vi "ME_acquire_10_DeltaForce_mod.vi"() -> ()   [LabVIEW 2015]
doc: "Use this template to build a producer/consumer design pattern. Use this template when you need to execute a process, such as data analysis, when a data source, such as a triggered acquisition, produces data at an uneven rate and you need to execute the process when the data becomes available."
uses:
  oxford_driver/Oxford Drivers/BUSGEN.LLB/OxfordAddress.ctl
  <vilib>/express/express arith-compare/Formula/XNode/ExpressFormulaBlockNode.xnode
  Mode.ctl
  <vilib>/Utility/file.llb/Write Delimited Spreadsheet (DBL).vi
  <vilib>/Analysis/NI_AALBase.lvlib
  <vilib>/Analysis/baseanly.llb/Mean (DBL).vi
panel:
  out "deltaUaux":dbl
  out "Actual Voltage (V)":dbl caption="Actual AuxV" step=0.1
  out "remaining elements":T1(array[cluster])
  in  "Stop":bool
  out "SaveSweep":bool=TRUE
  out "Measurement File_dn":path
  out "Measurement File_up":path
  out "Measurement File_average":path
  out "Actual Polarization":dbl
  in  "Reset IB?":bool
  in  "First?":bool
  in  "Save Period":dbl=1.0
  out "Averaged I(B)":dbl[][](array[numeric])
  out "P(uC/mm^2)":dbl[](array[numeric])
  in  "Sweep":bool
  out "P(B)":cluster{"yi":dbl[], dbl[]}(graph)
  out "Offset array":dbl[](array[numeric])
  in  "stop 2":bool
  in  "dB":dbl=0.005
  in  "Dwell Time (ms)":u32=1
  out "appended array":dbl[][](array[numeric])
  out "Actual B Field (T)":dbl
  out "Actual Temperature (K)":dbl
  out "Actual Current (pA)":dbl
  in  "Tab Control":T2(tab)
  in  "Max temperature (K)":dbl=20.0
  in  "Min Temperature (K)":dbl=4.5
  out "P(T)":cluster{"yi":dbl[], dbl[]}(graph)
  out "I(T)":cluster{dbl[], dbl[]}(graph)
  in  "Set temperature (K)":dbl=4.5
  in  "Temp Ramping Rate (K/min)":dbl=10.0
  in  "Heater Range":enum16{"Off", "Low", "Medium", "High"}(ring)
  in  "Heater On/Off":bool
  out "Setpoint Temperature (K)":dbl
  in  "FileName":string
  out "Step Temp":bool
  out "j":i32
  out "i":i32
  in  "Max Countl":i32
  in  "Record ALL":bool
  in  "Sweep Rate Array":dbl[](array[numeric])=[2.0, 1.0, 0.5, 0.1, 0.05, 9.0, 10.0, 11.0, 12.0]
  out "I(B) 3":cluster{dbl[], dbl[]}[](graph)
  in  "Go to Set":bool
  in  "Set Field (T)":dbl
  in  "Field To Zero":bool
  in  "Sweep Rate (T/min)":dbl=2.0 format="%.6f"
  in  "Min Field (T)":dbl
  in  "Max Field (T)":dbl=0.15
  out "Up/Down":bool
  out "I(B) /Averaged/ 2":cluster{"B array":dbl[], dbl[]}[](graph)
  in  "Temperature Array":dbl[](array[numeric])=[4.5, 5.0, 6.0, 7.0, 8.0, 9.0, 10.0, 11.0, 12.0]
  out "New":bool=TRUE
  out "Step Rate":bool
  out "Finished":bool=TRUE
  in  "Directory":string
  out "Wait (s)":dbl
  in  "secs to wait":dbl=180.0
  in  "Max count array":i32[](array[numeric])=[2, 1, 0, 0, 0, 9, 10, 11, 12]
  out "Target Field":dbl
  in  "Measure Noise":bool
  in  "Cycles":i32
  in  "maximum value":dbl=10.0 format="%0.2f"
  in  "minimum value":dbl=-10.0 format="%0.2f"
  in  "physical channels":tag="Dev1/ai1"
  out "PSD (pA/Hz^1/2) Peaks Removed":cluster{"f0":dbl, "df":dbl, "magnitude":dbl[]}(graph)
  out "PSD (pA/Hz^1/2)":cluster{"f0":dbl, "df":dbl, "magnitude":dbl[]}(graph)
  out "Current (pA) Filtered":waveform(dbl)(graph)
  out "Current (pA)":dbl[](graph)
  in  "Samples per channel":i32=1000
  in  "Rate":dbl=1000.0 format="%0.2f"
  in  "Cut-Off Frequency":dbl=100.0 caption="Lower Cut-Off"
  in  "Filter On":bool
  in  "Lock_in_Amplifier":refnum<visa-resource-name>="GPIB0::5::INSTR"
  out "Dc offset":dbl
  in  "Calibrate":bool
  in  "IV converter":refnum<visa-resource-name>="GPIB0::20::INSTR"
  in  "Magnetic Field":refnum<visa-resource-name>="GPIB0::21::INSTR"
  out "Time Lag":dbl=0.0500025749206543
  in  "Lake Shore":refnum<visa-resource-name>="GPIB0::11::INSTR"
  in  "Temp Refresh (s)":dbl=0.1
  in  "Sampling rate (Hz)":dbl=10.0
  in  "Gain (V/A)":dbl=1000000000.0
  in  "Sample area (mm^2)":dbl=3.9
  out "B_V":cluster{dbl[], "Best Linear Fit":dbl[]}[](graph)=[{[-0.00854253601, 0.00626134724, 0.0219834428, 0.0379117736, 0.0535871506, 0.0694316728, 0.0851615152, 0.100816481, 0.116478038, 0.132148461, 0.147876163, 0.16341701, 0.178976744, 0.194563632, 0.210251739, 0.225738944, 0.241298253, 0.256806034, 0.272344374, 0.287933477, 0.303494709, 0.318997125, 0.334591297, 0.350146681, 0.365618053, 0.380940961, 0.39666457, 0.412213675, 0.427724671, 0.443221444, 0.458760641, 0.474360042, 0.489915118, 0.505330598, 0.520967119, 0.536347531, 0.551813711, 0.567441155, 0.582995861, 0.598507522, 0.614041988, 0.629563151, 0.645106262, 0.660611914, 0.676136149, 0.691553948, 0.7071244, 0.72262999, 0.738171137, 0.753700392, 0.76919513, 0.784778028, 0.800215944, 0.8156961, 0.831325434, 0.846852183, 0.862326812, 0.877819169, 0.893312568, 0.90888536, 0.924354789], "Best Linear Fit"=[0.0, 0.005, 0.01, 0.015, 0.02, 0.025, 0.03, 0.035, 0.04, 0.045, 0.05, 0.055, 0.06, 0.065, 0.07, 0.075, 0.08, 0.085, 0.09, 0.095, 0.1, 0.105, 0.11, 0.115, 0.12, 0.125, 0.13, 0.135, 0.14, 0.145, 0.15, 0.155, 0.16, 0.165, 0.17, 0.175, 0.18, 0.185, 0.19, 0.195, 0.2, 0.205, 0.21, 0.215, 0.22, 0.225, 0.23, 0.235, 0.24, 0.245, 0.25, 0.255, 0.26, 0.265, 0.27, 0.275, 0.28, 0.285, 0.29, 0.295, 0.3]}, {[-0.00854253601, 0.00626134724, 0.0219834428, 0.0379117736, 0.0535871506, 0.0694316728, 0.0851615152, 0.100816481, 0.116478038, 0.132148461, 0.147876163, 0.16341701, 0.178976744, 0.194563632, 0.210251739, 0.225738944, 0.241298253, 0.256806034, 0.272344374, 0.287933477, 0.303494709, 0.318997125, 0.334591297, 0.350146681, 0.365618053, 0.380940961, 0.39666457, 0.412213675, 0.427724671, 0.443221444, 0.458760641, 0.474360042, 0.489915118, 0.505330598, 0.520967119, 0.536347531, 0.551813711, 0.567441155, 0.582995861, 0.598507522, 0.614041988, 0.629563151, 0.645106262, 0.660611914, 0.676136149, 0.691553948, 0.7071244, 0.72262999, 0.738171137, 0.753700392, 0.76919513, 0.784778028, 0.800215944, 0.8156961, 0.831325434, 0.846852183, 0.862326812, 0.877819169, 0.893312568, 0.90888536, 0.924354789], "Best Linear Fit"=[-0.00022554388023060128, 0.004536267537808887, 0.009593430775915074, 0.014716931562355689, 0.01975906732634002, 0.024855610270593523, 0.029915265354287977, 0.03495083565949541, 0.03998852608757118, 0.045029068349812316, 0.05008803495326229, 0.055086897848955874, 0.060091835929837946, 0.06510550835596321, 0.07015173884687344, 0.07513334727738563, 0.08013814865293042, 0.08512637555172443, 0.0901244320467579, 0.09513881694893507, 0.10014423687592358, 0.10513073807087174, 0.11014675346564809, 0.1151502923271957, 0.12012680792099008, 0.1250555686413888, 0.1301132186920259, 0.13511473785283767, 0.14010399888730068, 0.14508868495702945, 0.1500870171143548, 0.15510471446726903, 0.16010815425765457, 0.16506669165212906, 0.17009632901003072, 0.1750435864450521, 0.18001843198211442, 0.1850451496356715, 0.19004847041199868, 0.1950379453501071, 0.20003475573578386, 0.20502728708357412, 0.21002687821664084, 0.21501442030211, 0.220007939788244, 0.2249672231113706, 0.22997560874002893, 0.23496313088260184, 0.23996209027618054, 0.24495722449359253, 0.24994125598600042, 0.2549536449902534, 0.25991939913989753, 0.2648987401917687, 0.26992606578200207, 0.2749203939204135, 0.2798979571595809, 0.2848812227804405, 0.2898648235706211, 0.2948739618827834, 0.2998498524919418]}]
  out "V_I":cluster{dbl[], "Best Linear Fit":dbl[]}[](graph)=[{[0.0, 0.035, 0.069, 0.104, 0.138, 0.173, 0.208, 0.242, 0.277, 0.311, 0.346, 0.38, 0.415, 0.45, 0.484, 0.519, 0.553, 0.588, 0.623, 0.657, 0.692, 0.726, 0.761, 0.796, 0.83, 0.865, 0.899, 0.934, 0.969, 1.003, 1.038, 1.072, 1.107, 1.141, 1.176, 1.211, 1.245, 1.28, 1.314, 1.349, 1.384, 1.418, 1.453, 1.487, 1.522, 1.557, 1.591, 1.626, 1.66, 1.695, 1.73, 1.764, 1.799, 1.833, 1.868, 1.902, 1.937, 1.972, 2.006, 2.041, 2.075], "Best Linear Fit"=[-0.00854253601, 0.00626134724, 0.0219834428, 0.0379117736, 0.0535871506, 0.0694316728, 0.0851615152, 0.100816481, 0.116478038, 0.132148461, 0.147876163, 0.16341701, 0.178976744, 0.194563632, 0.210251739, 0.225738944, 0.241298253, 0.256806034, 0.272344374, 0.287933477, 0.303494709, 0.318997125, 0.334591297, 0.350146681, 0.365618053, 0.380940961, 0.39666457, 0.412213675, 0.427724671, 0.443221444, 0.458760641, 0.474360042, 0.489915118, 0.505330598, 0.520967119, 0.536347531, 0.551813711, 0.567441155, 0.582995861, 0.598507522, 0.614041988, 0.629563151, 0.645106262, 0.660611914, 0.676136149, 0.691553948, 0.7071244, 0.72262999, 0.738171137, 0.753700392, 0.76919513, 0.784778028, 0.800215944, 0.8156961, 0.831325434, 0.846852183, 0.862326812, 0.877819169, 0.893312568, 0.90888536, 0.924354789]}, {[0.0, 0.035, 0.069, 0.104, 0.138, 0.173, 0.208, 0.242, 0.277, 0.311, 0.346, 0.38, 0.415, 0.45, 0.484, 0.519, 0.553, 0.588, 0.623, 0.657, 0.692, 0.726, 0.761, 0.796, 0.83, 0.865, 0.899, 0.934, 0.969, 1.003, 1.038, 1.072, 1.107, 1.141, 1.176, 1.211, 1.245, 1.28, 1.314, 1.349, 1.384, 1.418, 1.453, 1.487, 1.522, 1.557, 1.591, 1.626, 1.66, 1.695, 1.73, 1.764, 1.799, 1.833, 1.868, 1.902, 1.937, 1.972, 2.006, 2.041, 2.075], "Best Linear Fit"=[-0.007846580254753975, 0.007882153481927697, 0.02316149482613275, 0.03889022856281441, 0.054169569907019474, 0.06989830364370113, 0.08562703738038281, 0.10090637872458785, 0.11663511246126955, 0.1319144538054746, 0.14764318754215625, 0.1629225288863613, 0.17865126262304296, 0.19437999635972467, 0.2096593377039297, 0.22538807144061138, 0.24066741278481643, 0.25639614652149806, 0.27212488025817977, 0.2874042216023848, 0.3031329553390665, 0.31841229668327153, 0.3341410304199532, 0.3498697641566349, 0.3651491055008399, 0.3808778392375216, 0.39615718058172666, 0.4118859143184083, 0.42761464805509, 0.442893989399295, 0.45862272313597674, 0.4739020644801818, 0.48963079821686345, 0.5049101395610684, 0.5206388732977502, 0.5363676070344319, 0.5516469483786369, 0.5673756821153185, 0.5826550234595236, 0.5983837571962053, 0.6141124909328869, 0.629391832277092, 0.6451205660137737, 0.6603999073579787, 0.6761286410946604, 0.691857374831342, 0.7071367161755471, 0.7228654499122288, 0.7381447912564338, 0.7538735249931156, 0.7696022587297972, 0.7848816000740022, 0.8006103338106839, 0.815889675154889, 0.8316184088915707, 0.8468977502357756, 0.8626264839724573, 0.878355217709139, 0.893634559053344, 0.9093632927900257, 0.9246426341342309]}]
  out "B0 (T)":dbl=0.0025222449819540214
  out "B/V (T/V)":dbl=0.321659617116981
  out "I0 (A)":dbl=-0.007846580254753975
  out "V/I (Ohm)":dbl=0.44939239247661916
  in  "Offset?":bool
  in  "Magnet":bool
  in  "Ramp":bool=TRUE
  in  "Temp/Magnetic Field":bool
  out "index":i8
  out "Read?":bool
  out "Magnetic Field (T)":dbl[](array[numeric])
  out "Reset":bool
  out "Measured Current (pA)":dbl[](array[numeric])
  out "Elapsed Time (s)":dbl[](array[numeric])
  out "Start time":timestamp
  in  "Enum":T3=enum."Process"
  out "B array":dbl[](array[numeric])
  in  "dB (T)":dbl=0.0025
  in  "Counter":i8
  out "L magnet (H)":dbl
  out "R magnet (mOhm)":dbl
  out "Actual Current (R0)":dbl
  out "Actual Field (T)":dbl
  out "Temperature array":dbl[](array[numeric])
  in  "New Measurement File":bool
  out "Measurement File":path
  out "refnum out":refnum<file>
  in  "Measuring":bool
  in  "Measure /Pause":bool
  in  "stop":bool
  # "DeltaForce"
  # "Discrete"
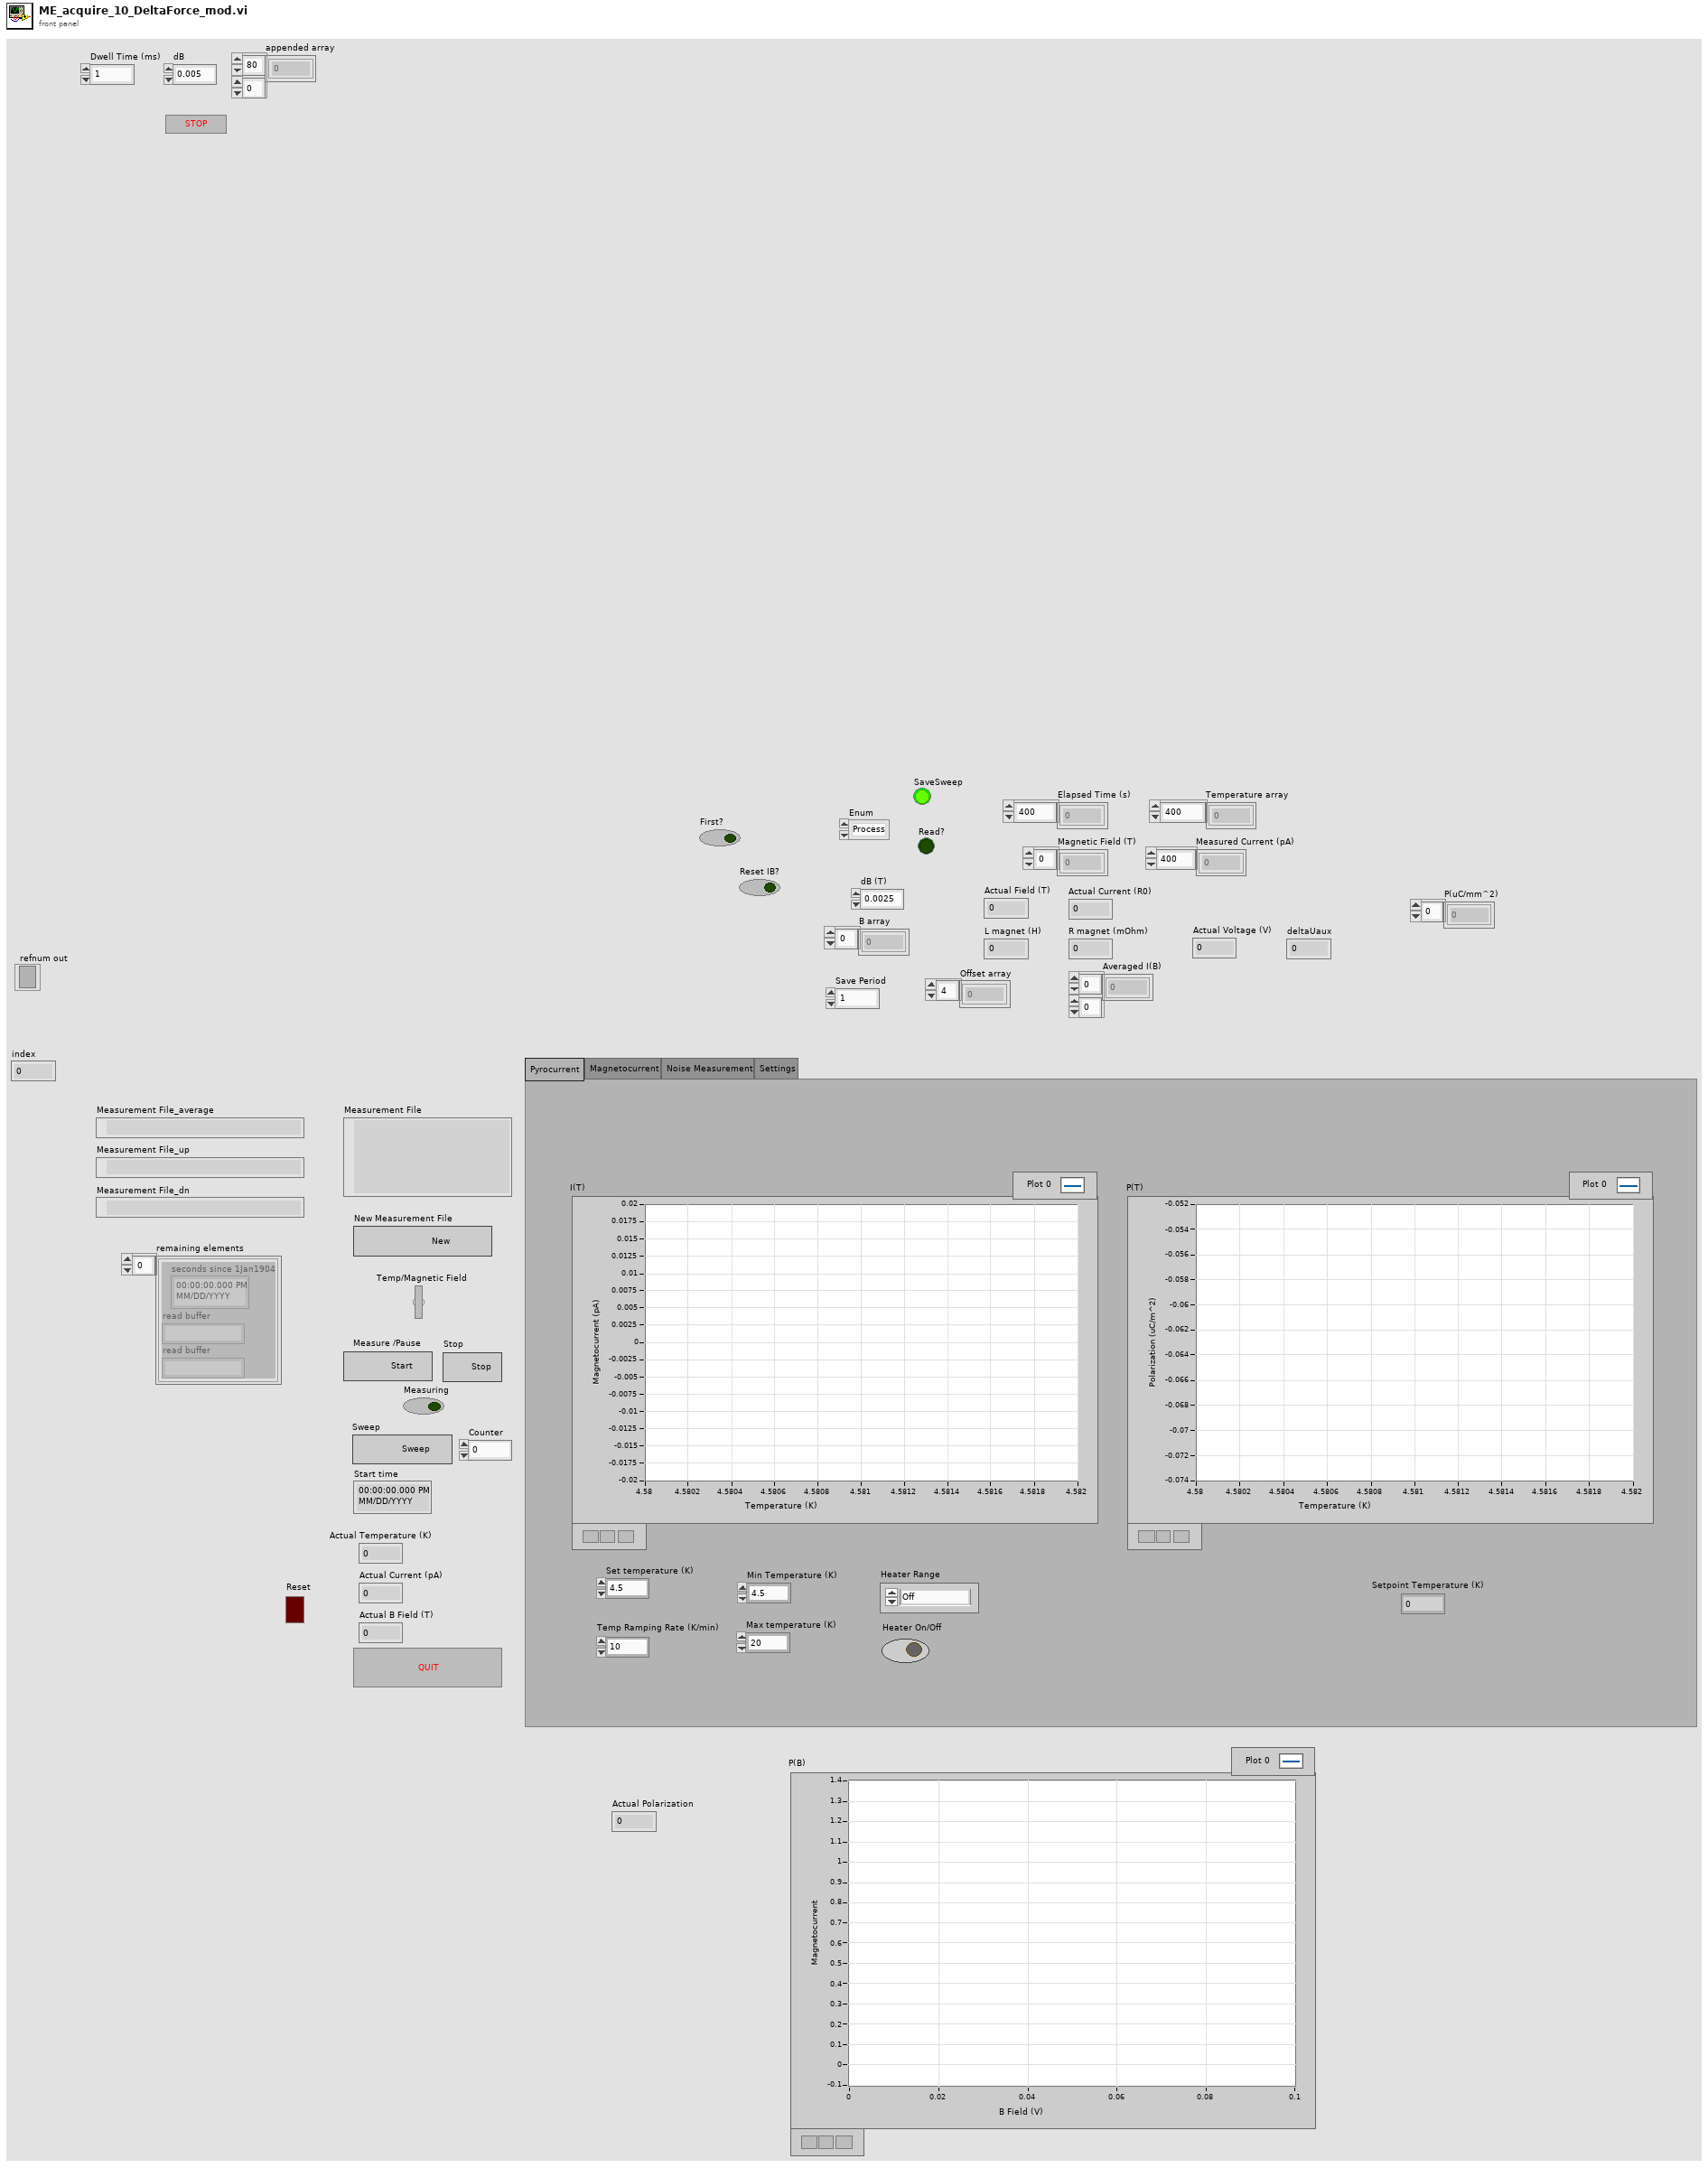
[diagram p1: front panel]
types:
  T1 = cluster{"seconds since 1Jan1904":timestamp, "read buffer":string, "read buffer":string}[]
  T2 = enum32{"Pyrocurrent", "Magnetocurrent", "Noise Measurement", "Settings"}
  T3 = typedef "Mode.ctl" = enum16{"Offset", "Process", "Sweep", "StepField", "Plot", "Save", "New", "Return", ""}
  T4 = enum16{"open", "replace", "create", "open or create", "replace or create", "replace or create with confirmation"}
  T5 = typedef "OxfordAddress.ctl" = cluster{"Com Port":i32, "ISOBUS Address":i32, "GPIB Address":i16, "Communication":enum16{"RS232", "ISOBUS", "GPIB", "Gateway"}}
  T6 = cluster{"seconds since 1Jan1904":timestamp, "read buffer":string, "read buffer":string}
  T7 = cluster{"B array":dbl[], "Averaged I(B) out":dbl[]}
  T8 = cluster{"B array":dbl[], "Averaged I(B) out":dbl[]}[]
  T9 = cluster{"I array out (A)":dbl[], "V array out (V)":dbl[]}
  T10 = cluster{"I array out (A)":dbl[], "Best Linear Fit":dbl[]}
  T11 = cluster{"V array out (V)":dbl[], "B array Out":dbl[]}
  T12 = cluster{"V array out (V)":dbl[], "Best Linear Fit 2":dbl[]}
  T13 = cluster{"I array out (A)":dbl[], "Best Linear Fit":dbl[]}[]
  T14 = cluster{"V array out (V)":dbl[], "Best Linear Fit 2":dbl[]}[]
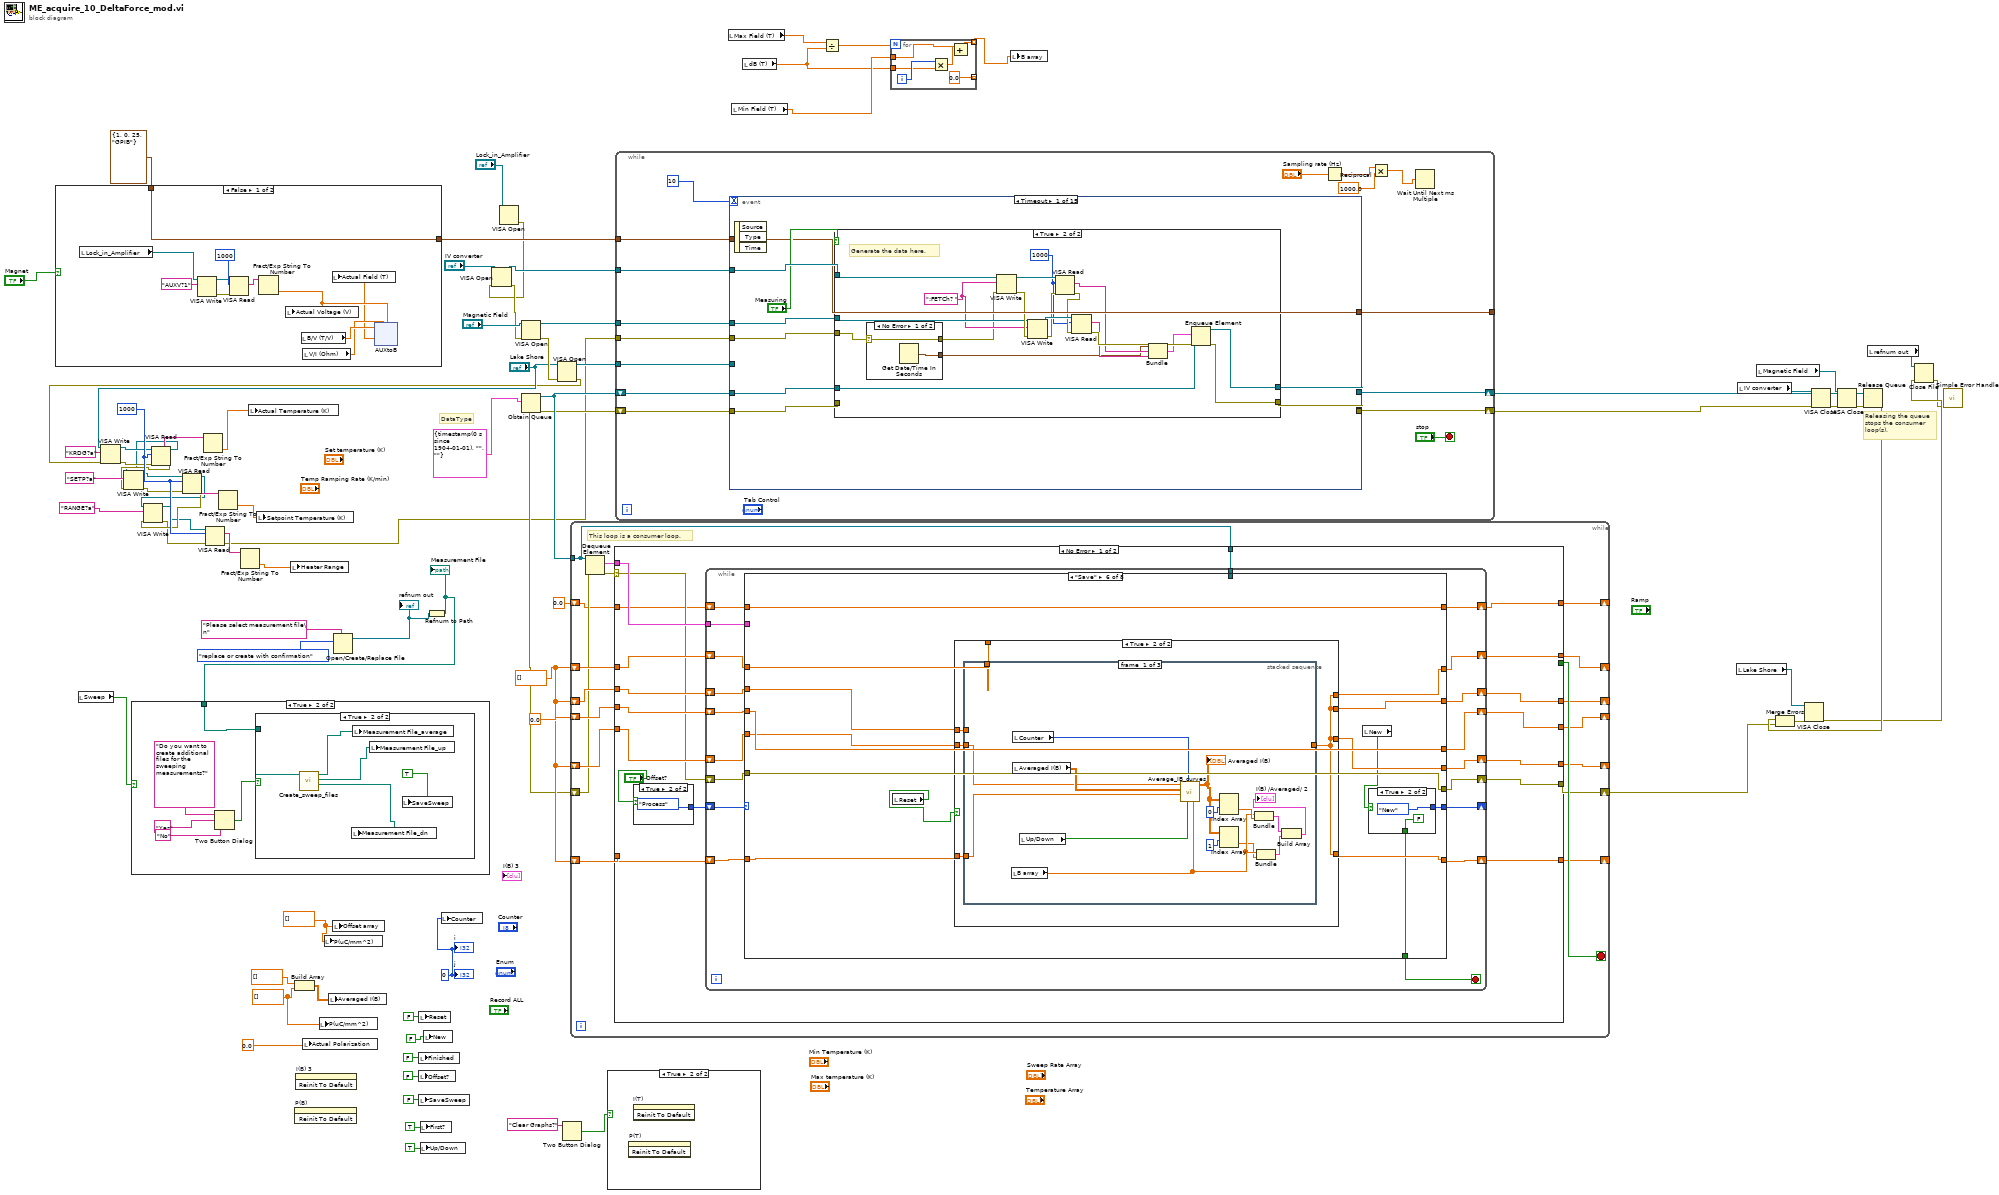
[diagram p0: block diagram]
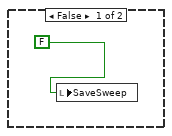
[diagram p4: hidden frame]
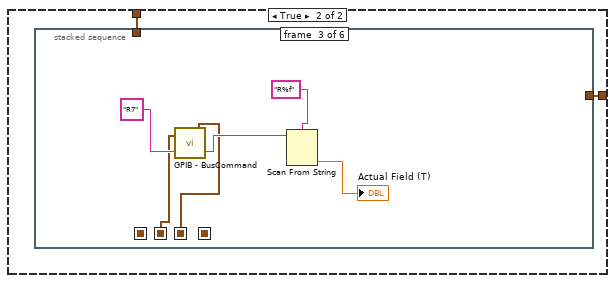
[diagram p5: hidden frame]
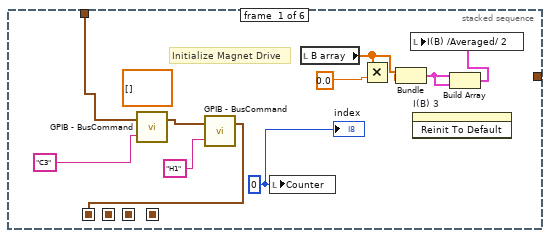
[diagram p6: hidden frame]
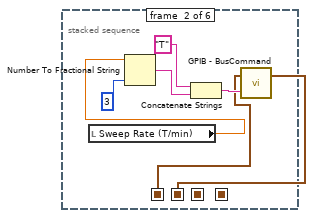
[diagram p7: hidden frame]
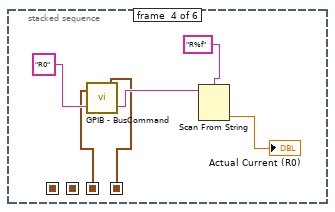
[diagram p8: hidden frame]
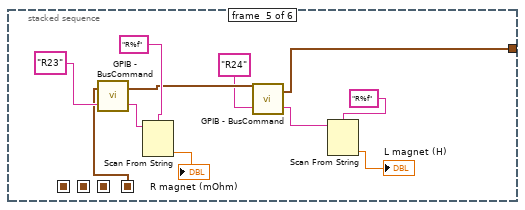
[diagram p9: hidden frame]
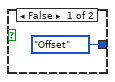
[diagram p11: hidden frame]
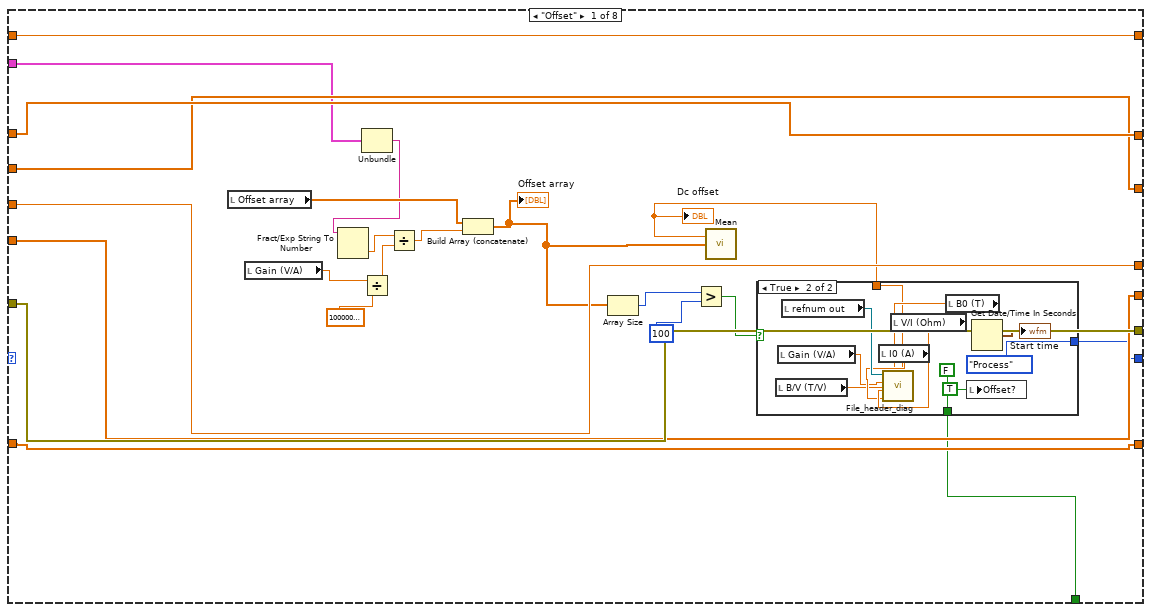
[diagram p12: hidden frame]
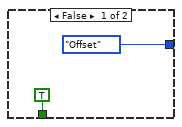
[diagram p13: hidden frame]
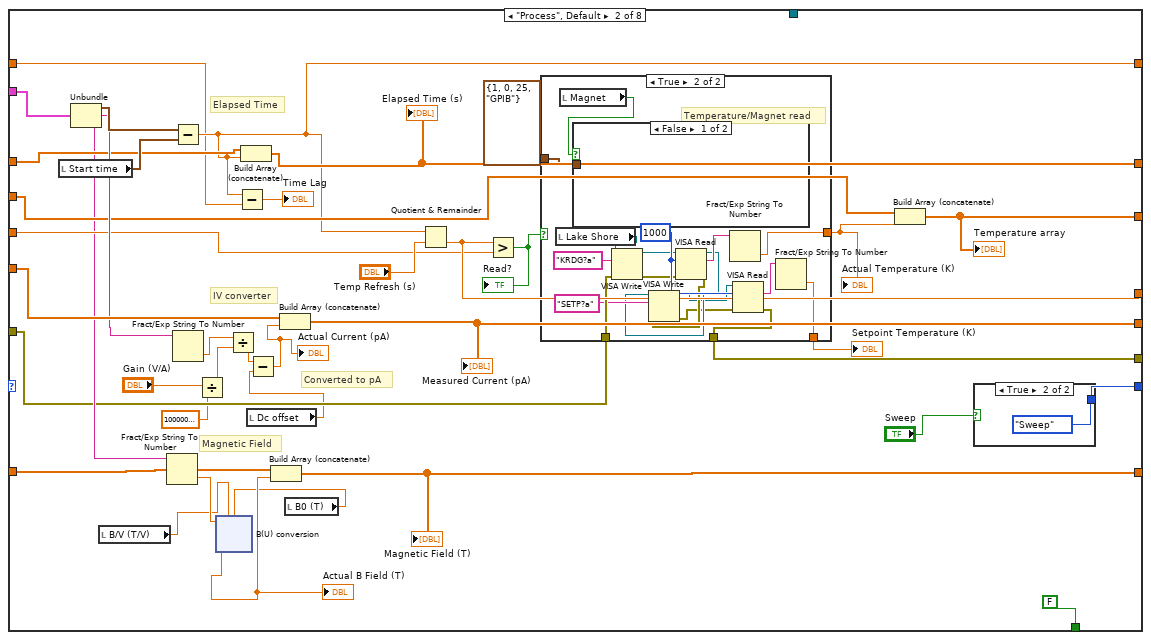
[diagram p14: hidden frame]
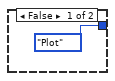
[diagram p15: hidden frame]
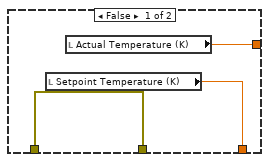
[diagram p16: hidden frame]
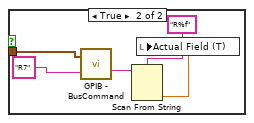
[diagram p17: hidden frame]
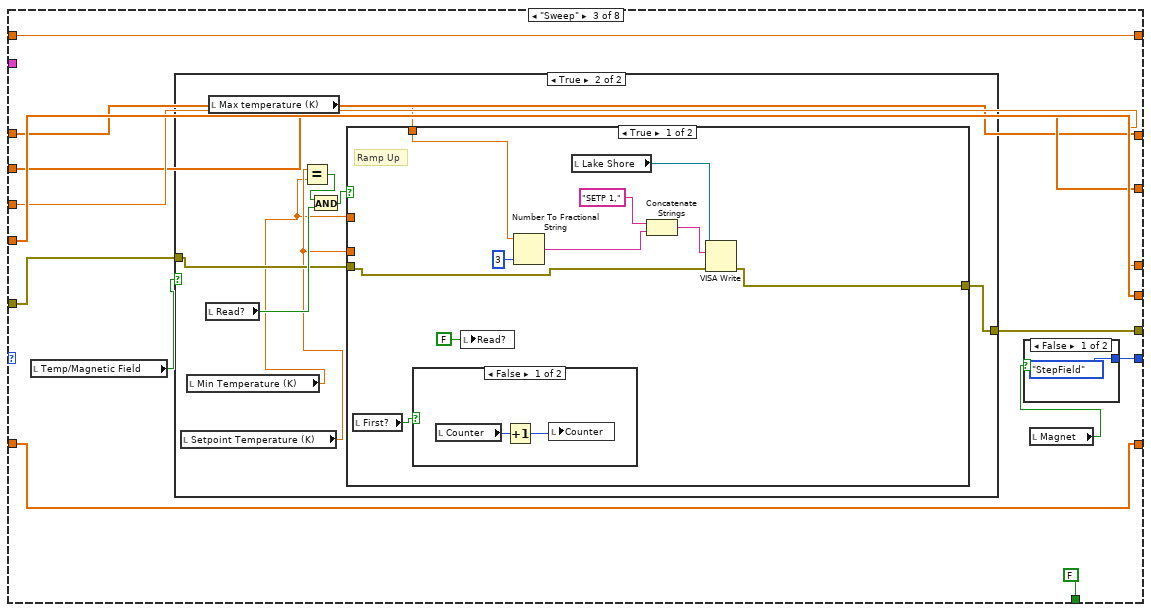
[diagram p18: hidden frame]
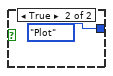
[diagram p19: hidden frame]
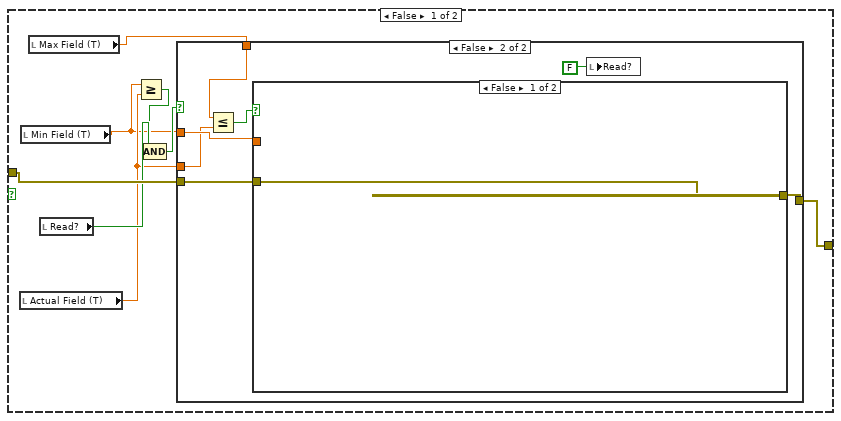
[diagram p20: hidden frame]
diagram:
  w19 = u32 1000 ("byte count")
  w30 = 0 ("j")
  w27 = dbl[] []
  w47 = dbl[] []
  w53 = dbl[] []
  # "DataType"
  # "Releasing the queue stops the consumer loop(s)."
  n1 = case shown="False" "Magnet" {
    tunnel: T5 {"Com Port"=1, "ISOBUS Address"=0, "GPIB Address"=25, "Communication"=enum."GPIB"} ("Address") -> [w90 w104]
    tunnel: [w90 w103] -> w59
    frame False {
      n2 = local read "Lock_in_Amplifier"() -> (w84:refnum<visa-resource-name>)
      n3 = VISA Write(VISA resource name=w84, write buffer="AUXV?1") -> (VISA resource name out=w85:refnum<visa-resource-name>, error out=w89:errorcluster)  [unwired: 1 in, 1 out]
      n4 = VISA Read(VISA resource name=w85, byte count=u32 1000, error in (no error)=w89) -> (read buffer=w88:string)  [unwired: 3 out]
      n5 = Fract/Exp String To Number(string=w88) -> (number=w81:dbl)  [unwired: 3 in, 1 out]
      n6 = local write "Actual Voltage (V)"(w81) -> ()
      n7 = local read "B/V (T/V)"() -> (w83:dbl)
      n8 = local read "V/I (Ohm)"() -> (w82:dbl)
      n9 = xnode "AUXtoB"("BpV"=w83, "Rm"=w82, "Aux"=w81) -> ("Result"=w80:dbl)  [unwired: 1 in, 1 out]
      n10 = local write "Actual Field (T)"(w80) -> ()
    }
    frame True {
      n11 = stacked-sequence {
        seq-local: [w112 _ _ _ _ _] -> [_ w117 _ _ _ _]
        seq-local: [_ w116 _ _ _ _] -> [_ _ w124 _ _ _]
        seq-local: [_ _ w123 _ _ _] -> [_ _ _ w130 _ _]
        seq-local: [_ _ _ w129 _ _] -> [_ _ _ _ w141 _]
        tunnel: w104 -> [w114 _ _ _ _ _]
        tunnel: [_ _ _ _ w139 _] -> w103
        frame #0 {
          (unwired) dbl[][] []
          w110 = i8 0 ("Counter")
          # "Initialize Magnet Drive"
          n12 = call "GPIB - BusCommand.vi"("Command"="C3", "Address"=w114) -> ("Address(thru)"=w113:T5)  [unwired: 1 out]
          n13 = call "GPIB - BusCommand.vi"("Command"="H1", "Address"=w113) -> ("Address(thru)"=w112:T5)  [unwired: 1 out]
          n14 = local write "Counter"(w110) -> ()
          n15 = local read "B array"() -> (w108:dbl[])
          n16 = Multiply(x=w108, y=0.0) -> (x*y=w107:dbl[])
          n17 = Bundle("B array"=w108, w107) -> (w106:cluster{"B array":dbl[], dbl[]})  [unwired: 1 in]
          n18 = invoke on="I(B) 3" class="XYGraph (strict)" method="Reinit To Default"() -> ()  [unwired: 3 in, 3 out]
          n19 = Build Array(w106, w106) -> (w105:cluster{"B array":dbl[], dbl[]}[])
          n20 = local write "I(B) /Averaged/ 2"(w105) -> ()
          "index" <- w110
        }
        frame #1 {
          n21 = local read "Sweep Rate (T/min)"() -> (w118:dbl)
          n22 = Number To Fractional String(number=w118, precision (6)=i16 3) -> (F-format string=w120:string)  [unwired: 2 in]
          n23 = Concatenate Strings("T" ("format string"), w120) -> (w119:string)
          n24 = call "GPIB - BusCommand.vi"("Command"=w119, "Address"=w117) -> ("Address(thru)"=w116:T5)  [unwired: 1 out]
        }
        frame #2 {
          n25 = call "GPIB - BusCommand.vi"("Command"="R7" ("format string"), "Address"=w124) -> ("Reply"=w128:string, "Address(thru)"=w123:T5)
          n26 = Scan From String(format string="R%f" ("remaining string"), input string=w128) -> (output 1=→"Actual Field (T)":dbl)  [unwired: 3 in, 3 out]
        }
        frame #3 {
          n27 = call "GPIB - BusCommand.vi"("Command"="R0" ("format string"), "Address"=w130) -> ("Reply"=w134:string, "Address(thru)"=w129:T5)
          n28 = Scan From String(format string="R%f" ("remaining string"), input string=w134) -> (output 1=→"Actual Current (R0)":dbl)  [unwired: 3 in, 3 out]
        }
        frame #4 {
          n29 = call "GPIB - BusCommand.vi"("Command"="R23" ("format string"), "Address"=w141) -> ("Reply"=w145:string, "Address(thru)"=w140:T5)
          n30 = Scan From String(format string="R%f" ("remaining string"), input string=w145) -> (output 1=→"R magnet (mOhm)":dbl)  [unwired: 3 in, 3 out]
          n31 = call "GPIB - BusCommand.vi"("Command"="R24" ("format string"), "Address"=w140) -> ("Reply"=w137:string, "Address(thru)"=w139:T5)
          n32 = Scan From String(format string="R%f" ("remaining string"), input string=w137) -> (output 1=→"L magnet (H)":dbl)  [unwired: 3 in, 3 out]
        }
        frame #5 {
        }
      }
    }
  }
  n33 = local read "Sweep"() -> (w35:bool)
  n34 = Build Array(dbl[] [], w27) -> (w45:dbl[][])
  n35 = invoke on="P(B)" class="XYGraph (strict)" method="Reinit To Default"() -> ()  [unwired: 3 in, 3 out]
  n36 = invoke on="I(B) 3" class="XYGraph (strict)" method="Reinit To Default"() -> ()  [unwired: 3 in, 3 out]
  n37 = local write "Actual Polarization"(0.0 ("Actual Polarization")) -> ()
  n38 = local write "P(uC/mm^2)"(w27) -> ()
  n39 = local write "P(uC/mm^2)"(w47) -> ()
  n40 = local write "Averaged I(B)"(w45) -> ()
  n41 = local write "Offset array"(w47) -> ()
  n42 = Open/Create/Replace File(prompt="Please select measurement file\n", operation (0:open)=T4."replace or create with confirmation") -> (refnum out=w56:refnum<file>)  [unwired: 4 in, 2 out]
  "refnum out" <- w56
  n43 = local write "Finished"(FALSE ("Finished")) -> ()
  n44 = local write "Offset?"(FALSE ("Offset?")) -> ()
  n45 = local write "Reset"(FALSE ("Reset")) -> ()
  n46 = local write "SaveSweep"(FALSE ("SaveSweep")) -> ()
  n47 = local write "First?"(TRUE ("First?")) -> ()
  n48 = local write "Up/Down"(TRUE ("Up/Down")) -> ()
  n49 = local write "New"(FALSE ("New")) -> ()
  n50 = Refnum to Path(1:w56) -> (0:w34:path)
  "Measurement File" <- w34
  n51 = case shown="True" w35 {
    tunnel: w34 -> [_ w146]
    frame False {
    }
    frame True {
      n52 = Two Button Dialog(message="Do you want to create additional files for the sweeping measurements?" ("string"), 1:"No" ("F button name (\"Cancel\")"), 2:"Yes" ("T button name (\"OK\")")) -> (T button?=w148:bool)
      n53 = case shown="True" w148 {
        tunnel: w146 -> [_ w156]
        frame False {
          n54 = local write "SaveSweep"(FALSE ("SaveSweep")) -> ()
        }
        frame True {
          n55 = call "Create_sweep_files.vi"("Measurement File"=w156) -> ("Path 3"=w153:path, "Path 2"=w154:path, "Path"=w155:path)  [unwired: 8 in]
          n56 = local write "Measurement File_dn"(w153) -> ()
          n57 = local write "Measurement File_average"(w155) -> ()
          n58 = local write "Measurement File_up"(w154) -> ()
          n59 = local write "SaveSweep"(TRUE) -> ()
        }
      }
    }
  }
  n60 = local write "Counter"(w30) -> ()
  n61 = VISA Open(VISA resource name="Lock_in_Amplifier") -> (error out=w2:errorcluster)  [unwired: 4 in, 1 out]
  n62 = VISA Open(error in (no error)=w2, VISA resource name="IV converter") -> (VISA resource name=w74:refnum<visa-resource-name>, error out=w76:errorcluster)  [unwired: 3 in]
  n63 = Obtain Queue(element data type=T6 {"seconds since 1Jan1904"=timestamp(0 s since 1904-01-01), "read buffer"="", "read buffer"=""} ("output cluster")) -> (queue out=w79:refnum<queue>, error out=w51:errorcluster)  [unwired: 4 in, 1 out]
  n64 = VISA Open(error in (no error)=w76, VISA resource name="Magnetic Field") -> (VISA resource name=w73:refnum<visa-resource-name>, error out=w54:errorcluster)  [unwired: 3 in]
  n65 = VISA Open(error in (no error)=w54, VISA resource name="Lake Shore") -> (VISA resource name=w49:refnum<visa-resource-name>, error out=w16:errorcluster)  [unwired: 3 in]
  n66 = VISA Write(VISA resource name="Lake Shore", write buffer="KRDG?a", error in (no error)=w16) -> (VISA resource name out=w13:refnum<visa-resource-name>, error out=w12:errorcluster)  [unwired: 1 out]
  n67 = VISA Read(VISA resource name=w13, byte count=w19, error in (no error)=w12) -> (VISA resource name out=w10:refnum<visa-resource-name>, read buffer=w24:string, error out=w11:errorcluster)  [unwired: 1 out]
  n68 = VISA Write(VISA resource name=w10, write buffer="SETP?a", error in (no error)=w11) -> (VISA resource name out=w9:refnum<visa-resource-name>, error out=w8:errorcluster)  [unwired: 1 out]
  n69 = VISA Read(VISA resource name=w9, byte count=w19, error in (no error)=w8) -> (VISA resource name out=w6:refnum<visa-resource-name>, read buffer=w23:string, error out=w7:errorcluster)  [unwired: 1 out]
  n70 = VISA Write(VISA resource name=w6, write buffer="RANGE?a", error in (no error)=w7) -> (VISA resource name out=w4:refnum<visa-resource-name>, error out=w5:errorcluster)  [unwired: 1 out]
  n71 = Fract/Exp String To Number(string=w24) -> (number=w22:dbl)  [unwired: 3 in, 1 out]
  n72 = VISA Read(VISA resource name=w4, byte count=w19, error in (no error)=w5) -> (read buffer=w18:string, error out=w15:errorcluster)  [unwired: 2 out]
  n73 = Fract/Exp String To Number(string=w23) -> (number=w21:dbl)  [unwired: 3 in, 1 out]
  n74 = Fract/Exp String To Number(string=w18) -> (number=w14:dbl)  [unwired: 3 in, 1 out]
  n75 = local write "Actual Temperature (K)"(w22) -> ()
  n76 = local write "Setpoint Temperature (K)"(w21) -> ()
  n77 = local write "Heater Range"(w14) -> ()
  n78 = Two Button Dialog(message="Clear Graphs?") -> (T button?=w29:bool)  [unwired: 2 in]
  n79 = while {
    tunnel: w79 -> [w157]
    shift-right: [w170] -> _
    shift-left: w53 -> [w169]
    shift-right: [w168] -> _
    shift-left: w53 -> [w167]
    shift-right: [w166] -> _
    shift-left: w53 -> [w165]
    shift-right: [w164] -> _
    shift-left: 0.0 -> [w163]
    shift-right: [w162] -> _
    shift-left: w53 -> [w161]
    shift-right: [w171] -> w64
    shift-left: w51 -> [w160]
    shift-right: [w159] -> _
    shift-left: 0.0 -> [w158]
    stop <- w172 stop-if-true
    # "This loop is a consumer loop."
    n80 = Dequeue Element(queue=w157, error in (no error)=w160) -> (element=w173:T6, error out=w174:errorcluster)  [unwired: 1 in, 2 out]
    n81 = case shown="No Error" w174 {
      selector: w174 -> [w180 w814]
      tunnel: w173 -> [w191 _]
      tunnel: [_ TRUE] -> w172
      tunnel: [w179 w814] -> w171
      tunnel: [w190 w813] -> w170
      tunnel: w169 -> [w189 w813]
      tunnel: [w188 w810] -> w168
      tunnel: w167 -> [w187 w810]
      tunnel: [w186 w809] -> w166
      tunnel: w165 -> [w185 w809]
      tunnel: [w184 w811] -> w164
      tunnel: w163 -> [w183 w811]
      tunnel: [w182 w812] -> w162
      tunnel: w161 -> [w181 w812]
      tunnel: [w178 w808] -> w159
      tunnel: w158 -> [w177 w808]
      tunnel: w157 -> [w175 _]
      frame No Error {
        n82 = case shown="True" "Offset?" {
          tunnel: [Mode."Offset" ("Enum") Mode."Process" ("Enum")] -> w192
          frame False {
          }
          frame True {
          }
        }
        n83 = while {
          shift-right: [w201] -> _
          shift-left: w192 -> [w213]
          tunnel: w191 -> [w212]
          shift-right: [w211] -> w190
          shift-left: w189 -> [w210]
          shift-right: [w203] -> w182
          shift-left: w181 -> [w202]
          shift-right: [w205] -> w184
          shift-left: w183 -> [w204]
          shift-right: [w209] -> w188
          shift-left: w187 -> [w208]
          shift-right: [w199] -> w179
          shift-left: w180 -> [w200]
          shift-right: [w207] -> w186
          shift-left: w185 -> [w206]
          shift-right: [w197] -> w178
          shift-left: w177 -> [w196]
          tunnel: w175 -> [w195]
          stop <- w198 stop-if-true
          n84 = case shown="\"Save\"" w213 {
            selector: w213 -> [_ _ _ _ _ _ _ w801]
            tunnel: w212 -> [w229 w285 _ _ _ _ _ _]
            tunnel: [w235 w282 w332 w447 w509 w582 w650 w806] -> w211
            tunnel: w210 -> [w235 w273 w332 w447 w509 w578 w650 w806]
            tunnel: [w230 w281 w335 w444 w511 w584 w648 w803] -> w209
            tunnel: w208 -> [w230 w280 w335 w444 w511 w579 w648 w803]
            tunnel: [w231 w277 w337 w442 w506 w585 w646 w800] -> w207
            tunnel: w206 -> [w231 w276 w337 w442 w506 w580 w646 w800]
            tunnel: [w233 w272 w334 w445 w507 w588 0.0 w804] -> w205
            tunnel: w204 -> [w233 w271 w334 w445 w507 w588 _ w804]
            tunnel: [w234 w268 w333 w446 w508 w583 w649 w805] -> w203
            tunnel: w202 -> [w234 w269 w333 w446 w508 w581 w649 w805]
            tunnel: [w218 w266 w330 Mode."Plot" ("Enum") Mode."Save" ("Enum") w589 Mode."Return" ("Enum") w801] -> w201
            tunnel: w200 -> [w232 w264 w339 w439 w514 w587 w642 w802]
            tunnel: [w232 w263 w338 w438 w514 w587 w641 w802] -> w199
            tunnel: [w214 FALSE FALSE FALSE FALSE w576 TRUE TRUE] -> w198
            tunnel: [w217 w260 w331 w440 w510 w586 0.0 w807] -> w197
            tunnel: w196 -> [w217 w259 w331 w440 w510 w586 _ w807]
            tunnel: w195 -> [_ _ _ _ _ _ w640 _]
            frame "Offset" {
              n85 = local read "Offset array"() -> (w223:dbl[])
              n86 = local read "Gain (V/A)"() -> (w227:dbl)
              n87 = Unbundle(w229) -> ("read buffer"=w216:string)  [unwired: 2 out]
              n88 = Fract/Exp String To Number(string=w216) -> (number=w228:dbl)  [unwired: 3 in, 1 out]
              n89 = Divide(x=w227, y=1000000000000.0) -> (x/y=w225:dbl)
              n90 = Divide(x=w228, y=w225) -> (x/y=w224:dbl)
              n91 = Build Array (concatenate)(w223, w224) -> (w219:dbl[])
              "Offset array" <- w219
              n92 = Array Size(array=w219) -> (size(s)=w222:i32)
              n93 = Greater?(x=w222, y=100) -> (0:w220:bool)
              n94 = call-poly <vilib>:"Mean.vi"("X"=w219) -> ("mean"=w215:dbl)  [unwired: 1 out]
              "Dc offset" <- w215
              n95 = case shown="True" w220 {
                tunnel: [Mode."Offset" ("Enum") Mode."Process" ("Enum")] -> w218
                tunnel: w215 -> [_ w240]
                tunnel: [TRUE FALSE] -> w214
                frame False {
                }
                frame True {
                  n96 = local read "B/V (T/V)"() -> (w241:dbl)
                  n97 = local read "Gain (V/A)"() -> (w242:dbl)
                  n98 = local read "refnum out"() -> (w246:refnum<file>)
                  n99 = local read "I0 (A)"() -> (w244:dbl)
                  n100 = local read "V/I (Ohm)"() -> (w245:dbl)
                  n101 = local read "B0 (T)"() -> (w243:dbl)
                  n102 = call "File_header_diag.vi"("OFFSET"=w240, "B0"=w243, "B/V"=w241, "I0"=w244, "V/I"=w245, "Gain"=w242, "Byte Stream File in"=w246) -> ()  [unwired: 5 in]
                  n103 = local write "Offset?"(TRUE ("Offset?")) -> ()
                  n104 = Get Date/Time In Seconds() -> (seconds since 1Jan1904=→"Start time":timestamp)
                }
              }
            }
            frame "Process", Default {
              # "Converted to pA"
              # "Magnetic Field"
              # "IV converter"
              # "Elapsed Time"
              n105 = local read "Start time"() -> (w283:timestamp)
              n106 = Unbundle(w285) -> ("seconds since 1Jan1904"=w284:timestamp, "read buffer"=w278:string, "read buffer"=w265:string)
              n107 = local read "B/V (T/V)"() -> (w255:dbl)
              n108 = Fract/Exp String To Number(string=w265) -> (number=w275:dbl)  [unwired: 3 in, 1 out]
              n109 = Subtract(x=w284, y=w283) -> (x-y=w260:dbl)
              n110 = Fract/Exp String To Number(string=w278) -> (number=w279:dbl)  [unwired: 3 in, 1 out]
              n111 = Divide(x="Gain (V/A)", y=1000000000000.0) -> (x/y=w258:dbl)
              n112 = Divide(x=w279, y=w258) -> (x/y=w253:dbl)
              n113 = Subtract(x=w260, y=w259) -> (x-y=→"Time Lag":dbl)
              n114 = Build Array (concatenate)(w273, w260) -> (w282:dbl[])
              "Elapsed Time (s)" <- w282
              n115 = local read "Dc offset"() -> (w251:dbl)
              n116 = Subtract(x=w253, y=w251) -> (x-y=w252:dbl)
              "Actual Current (pA)" <- w252
              n117 = Build Array (concatenate)(w280, w252) -> (w281:dbl[])
              "Measured Current (pA)" <- w281
              n118 = local read "B0 (T)"() -> (w254:dbl)
              n119 = xnode "B(U) conversion"("V"=w275, "BpV"=w255, "B0"=w254) -> ("Result"=w274:dbl)  [unwired: 1 in, 1 out]
              "Actual B Field (T)" <- w274
              n120 = Build Array (concatenate)(w276, w274) -> (w277:dbl[])
              "Magnetic Field (T)" <- w277
              n121 = Quotient & Remainder(x=w260, y="Temp Refresh (s)") -> (floor(x/y)=w272:dbl)  [unwired: 1 out]
              n122 = Greater?(x=w272, y=w271) -> (0:w270:bool)
              "Read?" <- w270
              n123 = case shown="True" w270 {
                tunnel: [w291 w308] -> w267
                tunnel: w264 -> [w292 w307]
                tunnel: [w292 w303] -> w263
                tunnel: T5 {"Com Port"=1, "ISOBUS Address"=0, "GPIB Address"=25, "Communication"=enum."GPIB"} ("Address") -> [_ w306]
                tunnel: [w290 w301] -> w249
                frame False {
                  n124 = local read "Setpoint Temperature (K)"() -> (w290:dbl)
                  n125 = local read "Actual Temperature (K)"() -> (w291:dbl)
                }
                frame True {
                  w302 = u32 1000 ("byte count")
                  # "Temperature/Magnet read"
                  n126 = local read "Lake Shore"() -> (w305:refnum<visa-resource-name>)
                  n127 = local read "Magnet"() -> (w293:bool)
                  n128 = case shown="False" w293 {
                    tunnel: w306 -> [_ w312]
                    frame False {
                    }
                    frame True {
                      n129 = call "GPIB - BusCommand.vi"("Command"="R7" ("format string"), "Address"=w312) -> ("Reply"=w313:string)  [unwired: 1 out]
                      n130 = Scan From String(format string="R%f" ("remaining string"), input string=w313) -> (output 1=w311:dbl)  [unwired: 3 in, 3 out]
                      n131 = local write "Actual Field (T)"(w311) -> ()
                    }
                  }
                  n132 = VISA Write(VISA resource name=w305, write buffer="KRDG?a", error in (no error)=w307) -> (VISA resource name out=w300:refnum<visa-resource-name>, error out=w298:errorcluster)  [unwired: 1 out]
                  n133 = VISA Read(VISA resource name=w300, byte count=w302, error in (no error)=w298) -> (VISA resource name out=w299:refnum<visa-resource-name>, read buffer=w309:string, error out=w297:errorcluster)  [unwired: 1 out]
                  n134 = VISA Write(VISA resource name=w299, write buffer="SETP?a", error in (no error)=w297) -> (VISA resource name out=w295:refnum<visa-resource-name>, error out=w296:errorcluster)  [unwired: 1 out]
                  n135 = Fract/Exp String To Number(string=w309) -> (number=w308:dbl)  [unwired: 3 in, 1 out]
                  n136 = VISA Read(VISA resource name=w295, byte count=w302, error in (no error)=w296) -> (read buffer=w294:string, error out=w303:errorcluster)  [unwired: 2 out]
                  n137 = Fract/Exp String To Number(string=w294) -> (number=w301:dbl)  [unwired: 3 in, 1 out]
                }
              }
              "Actual Temperature (K)" <- w267
              "Setpoint Temperature (K)" <- w249
              n138 = Build Array (concatenate)(w269, w267) -> (w268:dbl[])
              "Temperature array" <- w268
              n139 = case shown="True" "Sweep" {
                tunnel: [Mode."Plot" ("Enum") Mode."Sweep" ("Enum")] -> w266
                frame False {
                }
                frame True {
                }
              }
            }
            frame "Sweep" {
              n140 = local read "Temp/Magnetic Field"() -> (w329:bool)
              n141 = case shown="True" w329 {
                tunnel: w339 -> [w348 w405]
                tunnel: [w347 w404] -> w338
                frame False {
                  n142 = local read "Actual Field (T)"() -> (w343:dbl)
                  n143 = local read "Min Field (T)"() -> (w342:dbl)
                  n144 = local read "Max Field (T)"() -> (w349:dbl)
                  n145 = local read "Read?"() -> (w346:bool)
                  n146 = Greater Or Equal?(x=w342, y=w343) -> (x >= y?=w345:bool)
                  n147 = Compound Arithmetic op=AND(w345, w346) -> (w344:bool)
                  n148 = case shown="False" w344 {
                    tunnel: [w352 w388] -> w347
                    tunnel: w349 -> [w350 w387]
                    tunnel: w342 -> [_ w386]
                    tunnel: w343 -> [_ w384]
                    tunnel: w348 -> [w353 w383]
                    frame True {
                      # "Ramp Up"
                      n149 = case shown="True" "First?" {
                        tunnel: [TRUE ("Save") FALSE ("Save")] -> w356
                        tunnel: [w375 w379] -> w355
                        frame False {
                          n150 = local read "Counter"() -> (w378:i8)
                          n151 = local write "Actual Polarization"(0.0 ("Actual Polarization")) -> ()
                          n152 = Increment(x=w378) -> (x+1=w375:i8)
                          n153 = local write "Counter"(w375) -> ()
                        }
                        frame True {
                          n154 = local read "Counter"() -> (w379:i8)
                          n155 = local write "First?"(FALSE ("First?")) -> ()
                        }
                      }
                      "Reset" <- w356
                      n156 = local write "Read?"(FALSE ("Read?")) -> ()
                      n157 = local read "Record ALL"() -> (w351:bool)
                      n158 = case shown="True" w351 {
                        tunnel: w355 -> [_ w363]
                        tunnel: [FALSE w361] -> w354
                        frame False {
                        }
                        frame True {
                          n159 = Greater?(x=w363, y="Max Countl") -> (0:w361:bool)
                        }
                      }
                      n160 = case shown="False" w354 {
                        tunnel: w353 -> [w367 w374]
                        tunnel: [w366 w374] -> w352
                        tunnel: w350 -> [w365 _]
                        frame False {
                          n161 = local read "Magnet"() -> (w364:bool)
                          n162 = case shown="True" w364 {
                            tunnel: w367 -> [w368 w371]
                            tunnel: [w368 w370] -> w366
                            tunnel: w365 -> [_ w369]
                            frame False {
                            }
                            frame True {
                              n163 = call "Set_B.vi"("error in (no error)"=w371, "address string"="25", "Set Field (T)"=w369) -> ("error out"=w370:errorcluster)  [unwired: 8 in]
                            }
                          }
                          "Target Field" <- w365
                        }
                        frame True {
                          "New" <- TRUE
                        }
                      }
                      "Up/Down" <- FALSE ("Up/Down")
                    }
                    frame False {
                      n164 = Less Or Equal?(x=w387, y=w384) -> (x <= y?=w385:bool)
                      n165 = case shown="False" w385 {
                        tunnel: [w389 w393] -> w388
                        tunnel: w386 -> [_ w391]
                        tunnel: w383 -> [w389 w394]
                        frame False {
                        }
                        frame True {
                          # "Resetting at the end of every cycle"
                          # "Ramp Dn"
                          n166 = local write "Up/Down"(TRUE ("Up/Down")) -> ()
                          n167 = local read "Magnet"() -> (w390:bool)
                          n168 = local write "Target Field"(w391) -> ()
                          n169 = local write "Reset"(TRUE ("Reset")) -> ()
                          n170 = case shown="True" w390 {
                            tunnel: w394 -> [w396 w399]
                            tunnel: [w396 w398] -> w393
                            tunnel: w391 -> [_ w397]
                            frame False {
                            }
                            frame True {
                              n171 = call "Set_B.vi"("error in (no error)"=w399, "address string"="25", "Set Field (T)"=w397) -> ("error out"=w398:errorcluster)  [unwired: 8 in]
                            }
                          }
                        }
                      }
                      n172 = local write "Read?"(FALSE ("Read?")) -> ()
                    }
                  }
                }
                frame True {
                  n173 = local read "Setpoint Temperature (K)"() -> (w403:dbl)
                  n174 = local read "Min Temperature (K)"() -> (w402:dbl)
                  n175 = local read "Read?"() -> (w408:bool)
                  n176 = local read "Max temperature (K)"() -> (w401:dbl)
                  n177 = Equal?(x=w403, y=w402) -> (x = y?=w406:bool)
                  n178 = And(x=w406, y=w408) -> (x .and. y?=w407:bool)
                  n179 = case shown="True" w407 {
                    tunnel: [w410 w427] -> w404
                    tunnel: w401 -> [w409 w426]
                    tunnel: w402 -> [_ w425]
                    tunnel: w403 -> [_ w423]
                    tunnel: w405 -> [w411 w422]
                    frame True {
                      # "Ramp Up"
                      n180 = local read "First?"() -> (w417:bool)
                      n181 = case shown="False" w417 {
                        frame False {
                          n182 = local read "Counter"() -> (w420:i8)
                          n183 = Increment(x=w420) -> (x+1=w419:i8)
                          n184 = local write "Counter"(w419) -> ()
                        }
                        frame True {
                        }
                      }
                      n185 = local write "Read?"(FALSE ("Read?")) -> ()
                      n186 = Number To Fractional String(number=w409, precision (6)=i16 3) -> (F-format string=w414:string)  [unwired: 2 in]
                      n187 = local read "Lake Shore"() -> (w412:refnum<visa-resource-name>)
                      n188 = Concatenate Strings("SETP 1," ("write buffer"), w414) -> (w416:string)
                      n189 = VISA Write(VISA resource name=w412, write buffer=w416, error in (no error)=w411) -> (error out=w410:errorcluster)  [unwired: 2 out]
                    }
                    frame False {
                      n190 = Equal?(x=w426, y=w423) -> (x = y?=w424:bool)
                      n191 = case shown="True" w424 {
                        tunnel: [w428 w431] -> w427
                        tunnel: w425 -> [_ w430]
                        tunnel: w422 -> [w428 w432]
                        frame False {
                        }
                        frame True {
                          # "Ramp Dn"
                          n192 = local write "Up/Down"(TRUE ("Up/Down")) -> ()
                          n193 = Number To Fractional String(number=w430, precision (6)=i16 3) -> (F-format string=w434:string)  [unwired: 2 in]
                          n194 = local read "Lake Shore"() -> (w429:refnum<visa-resource-name>)
                          n195 = Concatenate Strings("SETP 1," ("write buffer"), w434) -> (w436:string)
                          n196 = VISA Write(VISA resource name=w429, write buffer=w436, error in (no error)=w432) -> (error out=w431:errorcluster)  [unwired: 2 out]
                        }
                      }
                      n197 = local write "Read?"(FALSE ("Read?")) -> ()
                    }
                  }
                }
              }
              n198 = local read "Magnet"() -> (w328:bool)
              n199 = case shown="False" w328 {
                tunnel: [Mode."StepField" ("Enum") Mode."Plot" ("Enum")] -> w330
                frame False {
                }
                frame True {
                }
              }
            }
            frame "StepField" {
              n200 = flat-sequence {
                tunnel: w439 -> [w455]
                tunnel: [w454] -> w438
                frame #0 {
                  # "Check if it is time to step Field"
                  n201 = local read "Sweep Rate (T/min)"() -> (w456:dbl)
                  n202 = local read "B/V (T/V)"() -> (w448:dbl)
                  n203 = local read "Time Lag"() -> (w452:dbl)
                  n204 = xnode "Sweep Delay"("SweepRate"=w456, "Resolution"=0.001 ("Voltage Step (V)"), "BpV"=w448) -> ("Result"=w453:dbl)  [unwired: 1 in, 1 out]
                  n205 = Divide(x=w452, y=w453) -> (x/y=w450:dbl)
                  n206 = Multiply(x=0.001 ("y"), y=w450) -> (x*y=w449:dbl)
                  "deltaUaux" <- w449
                  n207 = stacked-sequence {
                    tunnel: w455 -> [_ w480]
                    tunnel: [_ w479] -> w454
                    tunnel: w449 -> [w458 _]
                    frame #0 {
                      n208 = local read "Actual Voltage (V)"() -> (w463:dbl)
                      n209 = local read "Up/Down"() -> (w464:bool)
                      n210 = Add(x=w463, y=w458) -> (x+y=w460:dbl)
                      n211 = Subtract(x=w463, y=w458) -> (x-y=w459:dbl)
                      n212 = Select(t=w459, s=w464, f=w460) -> (s? t:f=w462:dbl)
                      "Actual Voltage (V)" <- w462
                      n213 = local read "V/I (Ohm)"() -> (w465:dbl)
                      n214 = local read "B/V (T/V)"() -> (w466:dbl)
                      n215 = xnode "AUXtoB"("BpV"=w466, "Rm"=w465, "Aux"=w462) -> ("Result"=w461:dbl)  [unwired: 1 in, 1 out]
                      n216 = local write "Actual Field (T)"(w461) -> ()
                    }
                    frame #1 {
                      n217 = local read "Actual Voltage (V)"() -> (w485:dbl)
                      n218 = local read "Lock_in_Amplifier"() -> (w481:refnum<visa-resource-name>)
                      n219 = Format Into String(w485) -> (resulting string=w484:string)  [unwired: 3 in, 1 out]
                      n220 = Concatenate Strings("AUXV 1,", w484) -> (w482:string)
                      n221 = VISA Write(VISA resource name=w481, write buffer=w482, error in (no error)=w480) -> (error out=w479:errorcluster)  [unwired: 2 out]
                    }
                  }
                }
              }
            }
            frame "Plot" {
              # "dI"
              n222 = local read "P(uC/mm^2)"() -> (w499:dbl[])
              n223 = local read "Actual Polarization"() -> (w498:dbl)
              n224 = local read "Actual Current (pA)"() -> (w500:dbl)
              n225 = local read "Time Lag"() -> (w512:dbl)
              n226 = Multiply(x=w500, y=w512) -> (x*y=w504:dbl)
              n227 = Divide(x=w504, y="Sample area (mm^2)") -> (x/y=w503:dbl)
              n228 = Add(x=w503, y=w498) -> (x+y=w502:dbl)
              "Actual Polarization" <- w502
              n229 = local read "Temp/Magnetic Field"() -> (w513:bool)
              n230 = Build Array (concatenate)(w499, w502) -> (→"P(uC/mm^2)":dbl[])
              n231 = case shown="True" w513 {
                tunnel: w510 -> [_ w573]
                tunnel: w507 -> [_ w555]
                tunnel: w502 -> [w520 w556]
                frame False {
                  # "Magnetic Field plotting"
                  n232 = local read "Up/Down"() -> (w525:bool)
                  n233 = local read "Actual B Field (T)"() -> (w522:dbl)
                  n234 = case shown="False" w525 {
                    frame True {
                      # "Down"
                      n235 = local read "I(B) 3"() -> (w535:cluster{dbl[], dbl[]}[])
                      n236 = local read "I(B) 3"() -> (w539:cluster{dbl[], dbl[]}[])
                      n237 = Index Array(array=w535, index=1) -> (element=w533:cluster{dbl[], dbl[]})
                      n238 = Unbundle(w533) -> (w532:dbl[], w531:dbl[])
                      n239 = Index Array(array=w539, index=i8 0 ("t")) -> (element=w536:cluster{dbl[], dbl[]})
                      n240 = local read "Actual Current (pA)"() -> (w528:dbl)
                      n241 = local read "Actual B Field (T)"() -> (w527:dbl)
                      n242 = Build Array (concatenate)(w532, w527) -> (w530:dbl[])
                      n243 = Build Array (concatenate)(w531, w528) -> (w529:dbl[])
                      n244 = Bundle(w530, w529) -> (w526:cluster{dbl[], dbl[]})  [unwired: 1 in]
                      n245 = Build Array(w536, w526) -> (w537:cluster{dbl[], dbl[]}[])
                      n246 = local write "I(B) 3"(w537) -> ()
                    }
                    frame False {
                      # "Up"
                      n247 = local read "I(B) 3"() -> (w551:cluster{dbl[], dbl[]}[])
                      n248 = local read "I(B) 3"() -> (w553:cluster{dbl[], dbl[]}[])
                      n249 = Index Array(array=w551, index=0) -> (element=w549:cluster{dbl[], dbl[]})
                      n250 = Unbundle(w549) -> (w548:dbl[], w547:dbl[])
                      n251 = Index Array(array=w553, index=i8 1 ("t")) -> (element=w541:cluster{dbl[], dbl[]})
                      n252 = local read "Actual B Field (T)"() -> (w543:dbl)
                      n253 = local read "Actual Current (pA)"() -> (w542:dbl)
                      n254 = Build Array (concatenate)(w548, w543) -> (w546:dbl[])
                      n255 = Build Array (concatenate)(w547, w542) -> (w545:dbl[])
                      n256 = Bundle(w546, w545) -> (w544:cluster{dbl[], dbl[]})  [unwired: 1 in]
                      n257 = Build Array(w544, w541) -> (w540:cluster{dbl[], dbl[]}[])
                      n258 = local write "I(B) 3"(w540) -> ()
                    }
                  }
                  n259 = local read "P(B)"() -> (w524:cluster{"yi":dbl[], dbl[]})
                  n260 = Unbundle(w524) -> ("yi"=w523:dbl[], w521:dbl[])
                  n261 = Build Array (concatenate)(w523, w522) -> (w519:dbl[])
                  n262 = Build Array (concatenate)(w521, w520) -> (w518:dbl[])
                  n263 = Bundle(w519, w518) -> (→"P(B)":cluster{dbl[], dbl[]})  [unwired: 1 in]
                }
                frame True {
                  # "Temperature plotting"
                  n264 = Quotient & Remainder(x=w573, y="Save Period") -> (x-y*floor(x/y)=w554:dbl)  [unwired: 1 out]
                  n265 = Greater?(x=w555, y=w554) -> (0:w571:bool)
                  n266 = local read "Actual Temperature (K)"() -> (w558:dbl)
                  n267 = local read "Actual Current (pA)"() -> (w564:dbl)
                  n268 = local read "P(T)"() -> (w560:cluster{"yi":dbl[], dbl[]})
                  n269 = local read "I(T)"() -> (w570:cluster{dbl[], dbl[]})
                  n270 = case shown="True" w571 {
                    frame False {
                    }
                    frame True {
                      n271 = local write "Reset"(TRUE) -> ()
                    }
                  }
                  n272 = Unbundle(w560) -> ("yi"=w561:dbl[], w557:dbl[])
                  n273 = Unbundle(w570) -> (w568:dbl[], w567:dbl[])
                  n274 = Build Array (concatenate)(w561, w558) -> (w562:dbl[])
                  n275 = Build Array (concatenate)(w557, w556) -> (w563:dbl[])
                  n276 = Build Array (concatenate)(w568, w558) -> (w566:dbl[])
                  n277 = Build Array (concatenate)(w567, w564) -> (w565:dbl[])
                  n278 = Bundle(w566, w565) -> (→"I(T)":cluster{dbl[], dbl[]})  [unwired: 1 in]
                  n279 = Bundle(w562, w563) -> (→"P(T)":cluster{dbl[], dbl[]})  [unwired: 1 in]
                }
              }
            }
            frame "Save" {
              n280 = local read "Reset"() -> (w575:bool)
              n281 = case shown="True" w575 {
                tunnel: w580 -> [w597 w599]
                tunnel: [w597 w602] -> w585
                tunnel: w579 -> [w596 w600]
                tunnel: [w596 w602] -> w584
                tunnel: w581 -> [w595 w601]
                tunnel: [w595 w602] -> w583
                tunnel: [w594 w602] -> w582
                tunnel: w578 -> [w594 w598]
                frame False {
                }
                frame True {
                  n282 = stacked-sequence {
                    tunnel: [_ _ w639] -> w602
                    tunnel: w601 -> [_ w628 _]
                    tunnel: w600 -> [w613 w626 _]
                    tunnel: w599 -> [w614 w627 _]
                    tunnel: w598 -> [_ w624 _]
                    frame #0 {
                      n283 = local read "B array"() -> (w604:dbl[])
                      n284 = local read "Counter"() -> (w612:i8)
                      n285 = local read "Averaged I(B)"() -> (w616:dbl[][])
                      n286 = local read "Up/Down"() -> (w615:bool)
                      n287 = call "Average_IB_curves.vi"("B array"=w604, "Up/Down"=w615, "Counter"=w612, "B in"=w614, "Averaged I(B) In"=w616, "I in"=w613) -> ("Averaged I(B) out"=w607:dbl[][])  [unwired: 5 in]
                      "Averaged I(B)" <- w607
                      n288 = Index Array(array=w607, index (row)=0 ("disabled index (col)")) -> (element=w605:dbl[])  [unwired: 1 in]
                      n289 = Index Array(array=w607, index (row)=1 ("disabled index (col)")) -> (element=w603:dbl[])  [unwired: 1 in]
                      n290 = Bundle("B array"=w604, "Averaged I(B) out"=w605) -> (w611:T7)  [unwired: 1 in]
                      n291 = Bundle("B array"=w604, "Averaged I(B) out"=w603) -> (w610:T7)  [unwired: 1 in]
                      n292 = Build Array(w611, w610) -> (→"I(B) /Averaged/ 2":T8)
                    }
                    frame #1 {
                      # "Save and Reset"
                      n293 = local read "Temp/Magnetic Field"() -> (w617:bool)
                      n294 = local read "Measurement File"() -> (w619:path)
                      n295 = local read "P(uC/mm^2)"() -> (w625:dbl[])
                      n296 = Build Array(w628, w627, w626, w624, w625) -> (w618:dbl[][])
                      n297 = case shown="False" w617 {
                        tunnel: w619 -> [_ _]
                        tunnel: w618 -> [w633 _]
                        frame False {
                          n298 = local read "Up/Down"() -> (w631:bool)
                          n299 = case shown="False" w631 {
                            tunnel: [w636 w637] -> w630
                            frame False {
                              n300 = local read "Measurement File_dn"() -> (w636:path)
                            }
                            frame True {
                              n301 = local read "Measurement File_up"() -> (w637:path)
                            }
                          }
                          n302 = call-poly <vilib>:"Write Delimited Spreadsheet.vi"("file path (dialog if empty)"=w630, "format (%.3f)"="%.5g", "2D data"=w633, "append to file? (F)"=TRUE ("transpose? (F)"), "transpose? (F)"=FALSE ("append to file? (F)")) -> ()  [unwired: 9 in, 2 out]
                        }
                        frame True {
                        }
                      }
                      n303 = case shown="False" "Reset IB?" {
                        frame False {
                        }
                        frame True {
                          n304 = local read "Up/Down"() -> (w638:bool)
                          n305 = case shown="False" w638 {
                            frame False {
                              n306 = invoke on="I(B) 3" class="XYGraph (strict)" method="Reinit To Default"() -> ()  [unwired: 3 in, 3 out]
                            }
                            frame True {
                            }
                          }
                        }
                      }
                      n307 = call-poly <vilib>:"Write Delimited Spreadsheet.vi"("file path (dialog if empty)"=w619, "format (%.3f)"="%.5g", "2D data"=w618, "append to file? (F)"=TRUE, "transpose? (F)"=TRUE) -> ()  [unwired: 9 in, 2 out]
                      n308 = local write "Reset"(FALSE ("Save")) -> ()
                    }
                    frame #2 {
                      w639 = dbl[] []
                      n309 = local write "P(uC/mm^2)"(w639) -> ()
                    }
                  }
                }
              }
              n310 = local read "New"() -> (w577:bool)
              n311 = case shown="True" w577 {
                tunnel: [Mode."Return" ("Enum") Mode."New" ("Enum")] -> w589
                tunnel: [TRUE FALSE] -> w576
                frame False {
                }
                frame True {
                }
              }
            }
            frame "New" {
              n312 = stacked-sequence {
                seq-local: [_ _ _ _ w733 _ _] -> [_ _ _ _ _ w742 _]
                seq-local: [_ _ w687 _ _ _ _] -> [_ _ _ _ w732 _ _]
                tunnel: T5 {"Com Port"=1, "ISOBUS Address"=0, "GPIB Address"=25, "Communication"=enum."GPIB"} ("Address") -> [_ _ w686 w727 _ _ _]
                tunnel: w642 -> [_ _ w688 _ _ w743 _]
                tunnel: [_ _ _ _ _ w745 _] -> w641
                tunnel: w640 -> [_ w667 _ _ _ _ _]
                frame #0 {
                  # "Save averages"
                  n313 = local read "Measurement File_average"() -> (w655:path)
                  n314 = local read "I(B) /Averaged/ 2"() -> (w656:cluster{"B array":dbl[], dbl[]}[])
                  n315 = Index Array(array=w656, index=0) -> (element=w659:cluster{"B array":dbl[], dbl[]})
                  n316 = Index Array(array=w656, index=1) -> (element=w660:cluster{"B array":dbl[], dbl[]})
                  n317 = Unbundle(w659) -> ("B array"=w661:dbl[], w662:dbl[])
                  n318 = Unbundle(w660) -> ("B array"=w663:dbl[], w664:dbl[])
                  n319 = Build Array(w661, w662, w663, w664) -> (w665:dbl[][])
                  n320 = call-poly <vilib>:"Write Delimited Spreadsheet.vi"("file path (dialog if empty)"=w655, "format (%.3f)"="%.5g", "2D data"=w665, "append to file? (F)"=TRUE ("transpose? (F)"), "transpose? (F)"=TRUE ("append to file? (F)")) -> ()  [unwired: 9 in, 2 out]
                }
                frame #1 {
                  w673 = dbl[] []
                  w682 = dbl[] []
                  # "Reset Flags"
                  n321 = Get Date/Time In Seconds() -> (seconds since 1Jan1904=w683:timestamp)
                  n322 = local write "Up/Down"(TRUE ("Up/Down")) -> ()
                  n323 = local write "First?"(TRUE ("First?")) -> ()
                  n324 = local write "Offset?"(FALSE ("Offset?")) -> ()
                  n325 = local write "New"(FALSE ("New")) -> ()
                  n326 = local write "P(uC/mm^2)"(w682) -> ()
                  n327 = local write "Start time"(w683) -> ()
                  n328 = local write "Offset array"(w682) -> ()
                  n329 = local write "Actual Polarization"(0.0 ("Actual Polarization")) -> ()
                  n330 = local write "Up/Down"(TRUE ("Up/Down")) -> ()
                  n331 = local write "Reset"(FALSE ("Reset")) -> ()
                  n332 = local read "B array"() -> (w676:dbl[])
                  n333 = local write "Counter"(i8 0 ("Counter")) -> ()
                  n334 = invoke on="P(B)" class="XYGraph (strict)" method="Reinit To Default"() -> ()  [unwired: 3 in, 3 out]
                  n335 = invoke on="I(B) 3" class="XYGraph (strict)" method="Reinit To Default"() -> ()  [unwired: 3 in, 3 out]
                  n336 = Multiply(x=w676, y=0.0) -> (x*y=w677:dbl[])
                  n337 = Build Array(w673, w673) -> (w681:dbl[][])
                  n338 = Bundle("B array"=w676, w677) -> (w678:cluster{"B array":dbl[], dbl[]})  [unwired: 1 in]
                  n339 = local write "Averaged I(B)"(w681) -> ()
                  n340 = Build Array(w678, w678) -> (w679:cluster{"B array":dbl[], dbl[]}[])
                  n341 = local write "I(B) /Averaged/ 2"(w679) -> ()
                  n342 = local write "Measuring"(FALSE ("Measuring")) -> ()
                  n343 = Flush Queue(queue=w667) -> (remaining elements=→"remaining elements":T1)  [unwired: 1 in, 2 out]
                }
                frame #2 {
                  # "Step"
                  n344 = local read "Sweep Rate Array"() -> (w692:dbl[])
                  n345 = local read "j"() -> (w693:i32)
                  n346 = Increment(x=w693) -> (x+1=w689:i32)
                  n347 = Array Size(array=w692) -> (size(s)=w691:i32)
                  n348 = Less?(x=w689, y=w691) -> (x < y?=w690:bool)
                  "Step Rate" <- w690
                  n349 = case shown="True" w690 {
                    tunnel: w689 -> [_ w720]
                    tunnel: w688 -> [w696 w719]
                    tunnel: [w695 w719] -> w687
                    tunnel: w686 -> [w694 _]
                    frame False {
                      # "Step Temp?"
                      n350 = local read "Temperature Array"() -> (w700:dbl[])
                      n351 = local read "i"() -> (w701:i32)
                      n352 = Increment(x=w701) -> (x+1=w698:i32)
                      n353 = local write "j"(0 ("f")) -> ()
                      n354 = Array Size(array=w700) -> (size(s)=w699:i32)
                      n355 = Less?(x=w698, y=w699) -> (x < y?=w697:bool)
                      "Step Temp" <- w697
                      n356 = case shown="False" w697 {
                        tunnel: w698 -> [_ w718]
                        tunnel: w696 -> [w706 w717]
                        tunnel: [w705 w717] -> w695
                        tunnel: w694 -> [w704 _]
                        frame False {
                          # "Heater OFF"
                          # "Finished"
                          n357 = local write "i"(0 ("i")) -> ()
                          n358 = stacked-sequence {
                            tunnel: w706 -> [w710 _ _]
                            tunnel: [w709 _ _] -> w705
                            tunnel: w704 -> [_ w714 w715]
                            frame #0 {
                              n359 = local read "Lake Shore"() -> (w711:refnum<visa-resource-name>)
                              n360 = VISA Write(VISA resource name=w711, write buffer="RANGE,1,0", error in (no error)=w710) -> (error out=w709:errorcluster)  [unwired: 2 out]
                            }
                            frame #1 {
                              n361 = call "ips_switchHeaterOff.vi"("Instrument address"=w714, "Rate"=2.0) -> ()  [unwired: 1 out]
                            }
                            frame #2 {
                              n362 = call "GPIB - BusCommand.vi"("Command"="H0", "Address"=w715) -> ()  [unwired: 2 out]
                            }
                          }
                          n363 = local write "Record ALL"(FALSE ("Record ALL")) -> ()
                          "Finished" <- TRUE
                        }
                        frame True {
                          n364 = local write "i"(w718) -> ()
                        }
                      }
                    }
                    frame True {
                      n365 = local write "j"(w720) -> ()
                    }
                  }
                }
                frame #3 {
                  # "Set rates"
                  n366 = local read "Sweep Rate Array"() -> (w726:dbl[])
                  n367 = local read "j"() -> (w725:i32)
                  n368 = local read "j"() -> (w723:i32)
                  n369 = Index Array(array=w726, index=w725) -> (element=w724:dbl)
                  n370 = Number To Fractional String(number=w724, precision (6)=i16 3) -> (F-format string=w730:string)  [unwired: 2 in]
                  n371 = Index Array(array="Max count array", index=w723) -> (element=w721:i32)
                  n372 = local write "Max Countl"(w721) -> ()
                  n373 = Concatenate Strings("T" ("format string"), w730) -> (w731:string)
                  n374 = call "GPIB - BusCommand.vi"("Command"=w731, "Address"=w727) -> ()  [unwired: 2 out]
                  n375 = local write "Sweep Rate (T/min)"(w724) -> ()
                }
                frame #4 {
                  # "Set temperature"
                  n376 = local read "Temperature Array"() -> (w736:dbl[])
                  n377 = local read "i"() -> (w735:i32)
                  n378 = Index Array(array=w736, index=w735) -> (element=w734:dbl)
                  n379 = local read "Lake Shore"() -> (w738:refnum<visa-resource-name>)
                  n380 = Number To Fractional String(number=w734, precision (6)=i16 3) -> (F-format string=w739:string)  [unwired: 2 in]
                  n381 = Concatenate Strings("SETP 1," ("write buffer"), w739) -> (w741:string)
                  n382 = VISA Write(VISA resource name=w738, write buffer=w741, error in (no error)=w732) -> (error out=w733:errorcluster)  [unwired: 2 out]
                }
                frame #5 {
                  n383 = local read "Finished"() -> (w744:bool)
                  n384 = case shown="False" w744 {
                    tunnel: [w758 w795] -> w745
                    tunnel: w743 -> [_ _]
                    tunnel: w742 -> [w755 w795]
                    frame False {
                      w753 = "_" ("string")
                      # "Wait, create Files"
                      n385 = local read "Temperature Array"() -> (w785:dbl[])
                      n386 = local read "Sweep Rate Array"() -> (w781:dbl[])
                      n387 = local read "i"() -> (w784:i32)
                      n388 = local read "j"() -> (w782:i32)
                      n389 = Index Array(array=w785, index=w784) -> (element=w783:dbl)
                      n390 = Index Array(array=w781, index=w782) -> (element=w750:dbl)
                      n391 = Round Toward -Infinity(1:w750) -> (0:w751:dbl)
                      n392 = Number To Fractional String(use system decimal point (T)=TRUE, number=w783, precision (6)=i16 1) -> (F-format string=w786:string)  [unwired: 1 in]
                      n393 = Subtract(x=w750, y=w751) -> (x-y=w752:dbl)
                      n394 = Equal To 0?(x=w752) -> (x = 0?=w749:bool)
                      n395 = Select(t=i16 0 ("precision (6)"), s=w749, f=i16 2 ("precision (6)")) -> (s? t:f=w746:i16)
                      n396 = Number To Fractional String(use system decimal point (T)=TRUE, number=w750, precision (6)=w746) -> (F-format string=w754:string)  [unwired: 1 in]
                      n397 = Concatenate Strings("Directory", "\\" ("string"), "FileName", w753, w786, "K" ("string"), w753, w754, "Tpm" ("string")) -> (w775:string)
                      n398 = Search and Replace String(replace all?=TRUE ("replace all? (F)"), input string=w775, search string=".", replace string="p" ("substring (\"\")"), error in=w755) -> (result string=w770:string, error out=w765:errorcluster)  [unwired: 3 in, 2 out]
                      n399 = local write "Step Rate"(FALSE ("Step Rate")) -> ()
                      n400 = Concatenate Strings(w770, ".txt" ("string")) -> (w769:string)
                      n401 = local read "Step Temp"() -> (w759:bool)
                      n402 = String To Path(string=w769) -> (path=w768:path)
                      n403 = Open/Create/Replace File(file path (use dialog)=w768, error in=w765, operation (0:open)=T4."open or create") -> (refnum out=w757:refnum<file>, error out=w758:errorcluster)  [unwired: 3 in, 1 out]
                      n404 = local write "refnum out"(w757) -> ()
                      n405 = Refnum to Path(1:w757) -> (0:w760:path)
                      n406 = call "Create_sweep_files.vi"("Measurement File"=w760) -> ("Path 3"=w763:path, "Path 2"=w762:path, "Path"=w761:path)  [unwired: 8 in]
                      n407 = local write "Measurement File"(w760) -> ()
                      n408 = case shown="True" w759 {
                        frame False {
                        }
                        frame True {
                          n409 = Get Date/Time In Seconds() -> (seconds since 1Jan1904=w788:timestamp)
                          n410 = local write "Step Temp"(FALSE ("Step Temp")) -> ()
                          n411 = while {
                            tunnel: w788 -> [w793]
                            stop <- w790 stop-if-true
                            n412 = Get Date/Time In Seconds() -> (seconds since 1Jan1904=w794:timestamp)
                            n413 = Subtract(x=w794, y=w793) -> (x-y=w792:dbl)
                            "Wait (s)" <- w792
                            n414 = Greater Or Equal?(x=w792, y="secs to wait") -> (x >= y?=w790:bool)
                          }
                        }
                      }
                      n415 = local write "Measurement File_dn"(w763) -> ()
                      n416 = local write "Measurement File_average"(w761) -> ()
                      n417 = local write "Measurement File_up"(w762) -> ()
                    }
                    frame True {
                    }
                  }
                }
                frame #6 {
                  n418 = local read "Finished"() -> (w796:bool)
                  n419 = case shown="True" w796 {
                    frame False {
                      n420 = local write "Measuring"(TRUE ("Measuring")) -> ()
                    }
                    frame True {
                      n421 = local write "Measure /Pause"(FALSE ("Measure /Pause")) -> ()
                    }
                  }
                }
              }
            }
            frame "Return" {
            }
          }
        }
      }
      frame Error {
        # "Return true for any case which should stop the loop."
      }
    }
  }
  n422 = case shown="True" w29 {
    frame False {
    }
    frame True {
      n423 = invoke on="P(T)" class="XYGraph (strict)" method="Reinit To Default"() -> ()  [unwired: 3 in, 3 out]
      n424 = invoke on="I(T)" class="XYGraph (strict)" method="Reinit To Default"() -> ()  [unwired: 3 in, 3 out]
    }
  }
  n425 = while {
    shift-right: [w827] -> w71
    shift-left: w51 -> [w828]
    shift-right: [w829] -> w78
    shift-left: w79 -> [w830]
    tunnel: w74 -> [w826]
    tunnel: w73 -> [w825]
    tunnel: w15 -> [w824]
    tunnel: [w818] -> _
    tunnel: w59 -> [w817]
    tunnel: w49 -> [w816]
    stop <- "stop" stop-if-true
    n426 = event shown="[0] Timeout" {
      selector: _ -> [_ _ _ _ _ _ _ _ _ _ _ _ _ _ _]
      dyn-events: _ -> [_ _ _ _ _ _ _ _ _ _ _ _ _ _ _]
      timeout: 10 -> [_ _ _ _ _ _ _ _ _ _ _ _ _ _ _]
      tunnel: w830 -> [w840 w872 w882 w896 w967 w971 w975 w1007 w1023 w1040 w1083 w1100 w1116 w1126 w1137]
      tunnel: [w839 w872 w882 w896 w967 w971 w975 w1007 w1023 w1040 w1083 w1100 w1116 w1126 w1137] -> w829
      tunnel: w828 -> [w838 w871 w881 w894 w966 w973 w977 w1008 w1022 w1039 w1084 w1102 w1120 w1130 w1139]
      tunnel: [w837 w871 w881 w893 w968 w973 w976 _ w1022 w1039 w1084 w1101 w1119 w1129 w1138] -> w827
      tunnel: w826 -> [w836 _ _ _ _ _ _ _ _ _ _ _ _ _ _]
      tunnel: w825 -> [w835 _ _ _ _ _ _ _ _ _ _ _ _ _ _]
      tunnel: w824 -> [w834 _ _ _ _ _ _ _ _ _ _ _ _ _ _]
      tunnel: [w832 w870 w880 w895 w969 w972 w974 w1006 w1021 w1038 w1082 w1099 w1117 w1127 _] -> w818
      tunnel: w817 -> [w832 w870 w883 w895 w969 w972 w974 w1006 w1021 w1038 w1082 w1099 w1117 w1127 _]
      tunnel: w816 -> [_ _ _ _ _ _ _ _ _ _ _ w1103 w1118 w1131 w1136]
      tunnel: [_ _ _ _ _ _ _ w1008 _ _ _ _ _ _ _] -> _
      event Timeout {
        n427 = event-data() -> ()  [unwired: 1 in, 3 out]
        n428 = case shown="True" "Measuring" {
          tunnel: w840 -> [w842 w861]
          tunnel: [w842 w860] -> w839
          tunnel: w838 -> [w841 _]
          tunnel: [w841 w859] -> w837
          tunnel: w836 -> [_ w852]
          tunnel: w835 -> [_ w851]
          tunnel: w834 -> [_ w846]
          frame False {
          }
          frame True {
            w849 = ":FETCh? " ("data")
            w853 = u32 1000 ("byte count")
            # "Generate the data here."
            n429 = case shown="No Error" w846 {
              selector: w846 -> [w863 w864]
              tunnel: [w863 w864] -> w845
              tunnel: [w862 _] -> w844
              frame No Error {
                n430 = Get Date/Time In Seconds() -> (seconds since 1Jan1904=w862:timestamp)
              }
              frame Error {
              }
            }
            n431 = VISA Write(VISA resource name=w852, write buffer=w849, error in (no error)=w845) -> (VISA resource name out=w858:refnum<visa-resource-name>, error out=w856:errorcluster)  [unwired: 1 out]
            n432 = VISA Write(VISA resource name=w851, write buffer=w849, error in (no error)=w856) -> (VISA resource name out=w857:refnum<visa-resource-name>, error out=w855:errorcluster)  [unwired: 1 out]
            n433 = VISA Read(VISA resource name=w858, byte count=w853, error in (no error)=w855) -> (read buffer=w847:string, error out=w854:errorcluster)  [unwired: 2 out]
            n434 = VISA Read(VISA resource name=w857, byte count=w853, error in (no error)=w854) -> (read buffer=w848:string, error out=w850:errorcluster)  [unwired: 2 out]
            n435 = Bundle("seconds since 1Jan1904"=w844, "read buffer"=w847, "read buffer"=w848) -> (w843:T6)  [unwired: 1 in]
            n436 = Enqueue Element(queue=w861, element=w843, error in (no error)=w850) -> (queue out=w860:refnum<queue>, error out=w859:errorcluster)  [unwired: 1 in, 1 out]
          }
        }
      }
      event "Max Field (T)": Value Change {
        n437 = event-data() -> ()  [unwired: 1 in, 6 out]
        n438 = Divide(x="Max Field (T)", y="dB (T)") -> (x/y=w867:dbl)
        n439 = for {
          N: w867 -> [_]
          tunnel: "dB (T)" -> [w877]
          tunnel: [w874] -> w866 mode=indexing
          tunnel: "Min Field (T)" -> [w875]
          tunnel: [0.0] -> _ mode=indexing
          i -> [w878]
          n440 = Multiply(x=w878, y=w877) -> (x*y=w876:dbl)
          n441 = Add(x=w876, y=w875) -> (x+y=w874:dbl)
        }
        "B array" <- w866
      }
      event "Sweep Rate (T/min)": Value Change {
        n442 = event-data() -> ("NewVal"=w884:dbl)  [unwired: 1 in, 5 out]
        n443 = local read "Magnet"() -> (w879:bool)
        n444 = case shown="False" w879 {
          tunnel: w884 -> [_ w891]
          tunnel: w883 -> [w885 w887]
          tunnel: [w885 w886] -> w880
          frame False {
          }
          frame True {
            n445 = Number To Fractional String(number=w891, precision (6)=i16 3) -> (F-format string=w889:string)  [unwired: 2 in]
            n446 = Concatenate Strings("T" ("format string"), w889) -> (w888:string)
            n447 = call "GPIB - BusCommand.vi"("Command"=w888, "Address"=w887) -> ("Address(thru)"=w886:T5)  [unwired: 1 out]
          }
        }
      }
      event "Field To Zero": Value Change {
        n448 = event-data() -> ()  [unwired: 1 in, 6 out]
        n449 = Two Button Dialog(message="Do you want to switch off the field?", 1:"No" ("F button name (\"Cancel\")"), 2:"Yes" ("T button name (\"OK\")")) -> (T button?=w900:bool)
        n450 = case shown="True" w900 {
          tunnel: w895 -> [_ w905]
          tunnel: w894 -> [w901 w903]
          tunnel: [w901 w902] -> w893
          frame False {
          }
          frame True {
            n451 = local read "Magnet"() -> (w904:bool)
            n452 = case shown="False" w904 {
              tunnel: w905 -> [_ w957]
              tunnel: w903 -> [w908 w954]
              tunnel: [w907 w954] -> w902
              frame False {
                n453 = local read "Lock_in_Amplifier"() -> (w906:refnum<visa-resource-name>)
                n454 = stacked-sequence {
                  seq-local: [w911 _] -> [_ w923]
                  seq-local: [w909 _] -> [_ w920]
                  tunnel: w908 -> [w913 _]
                  tunnel: [_ w926] -> w907
                  tunnel: w906 -> [w910 w921]
                  frame #0 {
                    n455 = VISA Write(VISA resource name=w910, write buffer="AUXV?1", error in (no error)=w913) -> (VISA resource name out=w917:refnum<visa-resource-name>, error out=w912:errorcluster)  [unwired: 1 out]
                    n456 = VISA Read(VISA resource name=w917, byte count=u32 1000, error in (no error)=w912) -> (read buffer=w914:string, error out=w911:errorcluster)  [unwired: 2 out]
                    n457 = Fract/Exp String To Number(string=w914) -> (number=w909:dbl)  [unwired: 3 in, 1 out]
                  }
                  frame #1 {
                    w929 = 0.001 ("Voltage Step (V)")
                    n458 = local read "Sweep Rate (T/min)"() -> (w928:dbl)
                    n459 = local read "V/I (Ohm)"() -> (w925:dbl)
                    n460 = local read "B/V (T/V)"() -> (w919:dbl)
                    n461 = xnode "Sweep Delay"("SweepRate"=w928, "Resolution"=w929, "BpV"=w919) -> ("Result"=w927:dbl)  [unwired: 1 in, 1 out]
                    n462 = call "Universal_Ramping.vi"("milliseconds to wait"=w927, "Initial Voltage (V)"=w920, "error in (no error)"=w923, "Voltage Step (V)"=w929, "Final Voltage (V)"=0.0, "VISA resource name"=w921) -> ("error out"=w926:errorcluster, "Actual Voltage (V)"=w918:dbl)  [unwired: 3 in, 1 out]
                    n463 = local write "Actual Voltage (V)"(w918) -> ()
                    n464 = xnode "AUXtoB"("BpV"=w919, "Rm"=w925, "Aux"=w918) -> ("Result"=w924:dbl)  [unwired: 1 in, 1 out]
                    n465 = local write "Actual B Field (T)"(w924) -> ()
                  }
                }
              }
              frame True {
                n466 = local read "Sweep Rate (T/min)"() -> (w956:dbl)
                n467 = call "ips_switchHeaterOff.vi"("Instrument address"=w957, "Rate"=w956) -> ("B"=w955:dbl)
                n468 = local write "Actual Field (T)"(w955) -> ()
              }
            }
          }
        }
      }
      event "Go to Set": Value Change {
        n469 = event-data() -> ()  [unwired: 1 in, 6 out]
        n470 = local read "V/I (Ohm)"() -> (w964:dbl)
        n471 = local read "B/V (T/V)"() -> (w963:dbl)
        n472 = local read "Lock_in_Amplifier"() -> (w960:refnum<visa-resource-name>)
        n473 = local read "Sweep Rate (T/min)"() -> (w962:dbl)
        n474 = local read "Magnet"() -> (w965:bool)
        n475 = call "Ramp_Field.vi"("Set Field (T) in"="Set Field (T)", "Sweep Rate (T/min)"=w962, "V/I (Ohm)"=w964, "error in (no error)"=w966, "Magnet"=w965, "B/V (T/V)"=w963, "VISA Refnum in"=w960) -> ("error out"=w968:errorcluster, "Actual Voltage (V)"=w958:dbl, "Set Field (T) out"=w961:dbl)  [unwired: 2 in]
        n476 = local write "Actual B Field (T)"(w961) -> ()
        n477 = local write "Actual Voltage (V)"(w958) -> ()
      }
      event "Measure /Pause": Value Change {
        n478 = event-data() -> ("NewVal"=w970:bool)  [unwired: 1 in, 5 out]
        n479 = local write "Measuring"(w970) -> ()
      }
      event "Stop": Value Change {
        n480 = event-data() -> ()  [unwired: 1 in, 6 out]
        n481 = local read "Measuring"() -> (w978:bool)
        n482 = case shown="True" w978 {
          tunnel: w977 -> [w979 w982]
          tunnel: [w979 w983] -> w976
          frame False {
          }
          frame True {
            w990 = FALSE ("Measuring")
            n483 = local read "SaveSweep"() -> (w991:bool)
            n484 = local write "Measuring"(w990) -> ()
            n485 = local write "Measure /Pause"(w990) -> ()
            n486 = local read "Lock_in_Amplifier"() -> (w984:refnum<visa-resource-name>)
            n487 = case shown="True" w991 {
              frame False {
              }
              frame True {
                n488 = local read "Measurement File_average"() -> (w1002:path)
                n489 = local read "I(B) /Averaged/ 2"() -> (w1001:cluster{"B array":dbl[], dbl[]}[])
                n490 = Index Array(array=w1001, index=0) -> (element=w998:cluster{"B array":dbl[], dbl[]})
                n491 = Index Array(array=w1001, index=1) -> (element=w997:cluster{"B array":dbl[], dbl[]})
                n492 = Unbundle(w998) -> ("B array"=w996:dbl[], w995:dbl[])
                n493 = Unbundle(w997) -> ("B array"=w994:dbl[], w993:dbl[])
                n494 = Build Array(w996, w995, w994, w993) -> (w992:dbl[][])
                n495 = call-poly <vilib>:"Write Delimited Spreadsheet.vi"("file path (dialog if empty)"=w1002, "format (%.3f)"="%.5g", "2D data"=w992, "append to file? (F)"=TRUE ("transpose? (F)"), "transpose? (F)"=TRUE ("append to file? (F)")) -> ()  [unwired: 9 in, 2 out]
              }
            }
            n496 = local read "V/I (Ohm)"() -> (w988:dbl)
            n497 = local read "Sweep Rate (T/min)"() -> (w987:dbl)
            n498 = local read "Set Field (T)"() -> (w989:dbl)
            n499 = local read "B/V (T/V)"() -> (w985:dbl)
            n500 = local read "Magnet"() -> (w986:bool)
            n501 = call "Ramp_Field.vi"("Set Field (T) in"=w989, "Sweep Rate (T/min)"=w987, "V/I (Ohm)"=w988, "error in (no error)"=w982, "Magnet"=w986, "B/V (T/V)"=w985, "VISA Refnum in"=w984) -> ("error out"=w983:errorcluster, "Actual Voltage (V)"=w980:dbl, "Set Field (T) out"=w981:dbl)  [unwired: 2 in]
            n502 = local write "Actual B Field (T)"(w981) -> ()
            n503 = local write "Actual Voltage (V)"(w980) -> ()
          }
        }
      }
      event "Sweep": Value Change {
        n504 = event-data() -> ("NewVal"=w1009:bool)  [unwired: 1 in, 5 out]
        n505 = case shown="True" w1009 {
          frame False {
          }
          frame True {
            n506 = local read "Measurement File"() -> (w1010:path)
            n507 = Two Button Dialog(message="Do you want to create additional files for the sweeping measurements?" ("string"), 1:"No" ("F button name (\"Cancel\")"), 2:"Yes" ("T button name (\"OK\")")) -> (T button?=w1012:bool)
            n508 = case shown="True" w1012 {
              tunnel: w1010 -> [_ w1017]
              frame False {
                n509 = local write "SaveSweep"(FALSE ("SaveSweep")) -> ()
              }
              frame True {
                n510 = call "Create_sweep_files.vi"("Measurement File"=w1017) -> ("Path 3"=→"Measurement File_dn":path, "Path 2"=→"Measurement File_up":path, "Path"=→"Measurement File_average":path)  [unwired: 8 in]
                "SaveSweep" <- TRUE
              }
            }
          }
        }
      }
      event "Measure Noise": Value Change {
        n511 = event-data() -> ("NewVal"=w1024:bool)  [unwired: 1 in, 5 out]
        n512 = case shown="True" w1024 {
          frame False {
          }
          frame True {
            n513 = local read "Gain (V/A)"() -> (w1029:dbl)
            n514 = call "Noise_measurement.vi"("Gain (V/A)"=w1029, "Cycles"="Cycles", "Lower Cut-Off"="Cut-Off Frequency", "minimum value"="minimum value", "Filter On"="Filter On", "maximum value"="maximum value", "physical channels"="physical channels", "rate"="Rate", "samples per channel"="Samples per channel") -> ("Current (pA) Filtered"=→"Current (pA) Filtered":waveform(dbl), "PSD (pA/Hz^1/2) Peaks Removed"=→"PSD (pA/Hz^1/2) Peaks Removed":cluster{"f0":dbl, "df":dbl, "magnitude":dbl[]}, "Current (pA)"=→"Current (pA)":dbl[], "PSD (pA/Hz^1/2)"=→"PSD (pA/Hz^1/2)":cluster{"f0":dbl, "df":dbl, "magnitude":dbl[]})  [unwired: 3 in]
          }
        }
      }
      event "Calibrate": Value Change {
        n515 = event-data() -> ()  [unwired: 1 in, 6 out]
        n516 = case shown="True" "Calibrate" {
          frame False {
          }
          frame True {
            w1044 = dbl[] []
            n517 = while {
              shift-right: [w1077] -> w1042
              shift-left: dbl[][] [] -> [w1076]
              shift-right: [w1060] -> _
              shift-left: w1044 -> [w1072]
              shift-right: [w1069] -> _
              shift-left: w1044 -> [w1071]
              shift-right: [w1059] -> _
              shift-left: w1044 -> [w1070]
              shift-right: [w1051] -> _
              shift-left: 0.0 ("Set Field out") -> [w1050]
              stop <- w1073 stop-if-true
              n518 = call "Calibtarion.vi"("Dwell Time (ms)"="Dwell Time (ms)", "V array in (V)"=w1072, "I array in (A)"=w1070, "Collected array in"=w1076, "B array in (T)"=w1071, "Set Field (T)"=w1050, "dB"="dB") -> ("Best Linear Fit"=w1061:dbl[], "appended array"=→"appended array":dbl[][], "slope"=→"B/V (T/V)":dbl, "V array out (V)"=w1060:dbl[], "Boolean"=w1075:bool, "I array out (A)"=w1059:dbl[], "intercept 2"=→"I0 (A)":dbl, "Collected array out"=w1077:dbl[][], "intercept"=→"B0 (T)":dbl, "B array Out"=w1069:dbl[], "slope 2"=→"V/I (Ohm)":dbl, "Best Linear Fit 2"=w1066:dbl[], "Set Field out"=w1051:dbl)
              n519 = Bundle("I array out (A)"=w1059, "V array out (V)"=w1060) -> (w1068:T9)  [unwired: 1 in]
              n520 = Bundle("I array out (A)"=w1059, "Best Linear Fit"=w1061) -> (w1062:T10)  [unwired: 1 in]
              n521 = Bundle("V array out (V)"=w1060, "B array Out"=w1069) -> (w1064:T11)  [unwired: 1 in]
              n522 = Bundle("V array out (V)"=w1060, "Best Linear Fit 2"=w1066) -> (w1065:T12)  [unwired: 1 in]
              n523 = Or(x=w1075, y="stop 2") -> (x .or. y?=w1073:bool)
              n524 = Build Array(w1068, w1062) -> (→"V_I":T13)
              n525 = Build Array(w1064, w1065) -> (→"B_V":T14)
            }
            n526 = flat-sequence {
              tunnel: w1042 -> [w1048]
              frame #0 {
                n527 = Two Button Dialog(message="Do you want to save calibration file?") -> (T button?=w1047:bool)  [unwired: 2 in]
                n528 = case shown="True" w1047 {
                  tunnel: w1048 -> [_ w1049]
                  frame False {
                  }
                  frame True {
                    n529 = call-poly <vilib>:"Write Delimited Spreadsheet.vi"("2D data"=w1049) -> ()  [unwired: 13 in, 2 out]
                  }
                }
              }
            }
          }
        }
      }
      event "New Measurement File": Value Change {
        n530 = event-data() -> ()  [unwired: 1 in, 6 out]
        n531 = local read "Sweep"() -> (w1079:bool)
        n532 = Open/Create/Replace File(prompt="Please select measurement file\n", operation (0:open)=T4."replace or create with confirmation") -> (refnum out=w1085:refnum<file>)  [unwired: 4 in, 2 out]
        n533 = local write "refnum out"(w1085) -> ()
        n534 = Refnum to Path(1:w1085) -> (0:w1080:path)
        n535 = case shown="True" w1079 {
          tunnel: w1080 -> [_ w1088]
          frame False {
          }
          frame True {
            n536 = Two Button Dialog(message="Do you want to create additional files for the sweeping measurements?" ("string"), 1:"No" ("F button name (\"Cancel\")"), 2:"Yes" ("T button name (\"OK\")")) -> (T button?=w1090:bool)
            n537 = case shown="False" w1090 {
              tunnel: w1088 -> [_ w1098]
              frame False {
                n538 = local write "SaveSweep"(FALSE ("SaveSweep")) -> ()
              }
              frame True {
                n539 = call "Create_sweep_files.vi"("Measurement File"=w1098) -> ("Path 3"=w1095:path, "Path 2"=w1096:path, "Path"=w1097:path)  [unwired: 8 in]
                n540 = local write "Measurement File_dn"(w1095) -> ()
                n541 = local write "Measurement File_average"(w1097) -> ()
                n542 = local write "Measurement File_up"(w1096) -> ()
                n543 = local write "SaveSweep"(TRUE) -> ()
              }
            }
          }
        }
        n544 = local write "Measurement File"(w1080) -> ()
        n545 = local write "Offset?"(FALSE ("Offset?")) -> ()
        n546 = local write "First?"(TRUE ("First?")) -> ()
      }
      event "Heater On/Off": Value Change {
        n547 = event-data() -> ()  [unwired: 1 in, 6 out]
        n548 = case shown="False" "Heater On/Off" {
          tunnel: w1103 -> [w1108 w1114]
          tunnel: w1102 -> [w1106 w1115]
          tunnel: [w1105 w1113] -> w1101
          frame False {
            n549 = VISA Write(VISA resource name=w1108, write buffer="RANGE,1,0", error in (no error)=w1106) -> (error out=w1105:errorcluster)  [unwired: 2 out]
          }
          frame True {
            n550 = Number To Decimal String(number="Heater Range") -> (decimal integer string=w1111:string)  [unwired: 1 in]
            n551 = Concatenate Strings("RANGE,1," ("write buffer"), w1111) -> (w1109:string)
            n552 = VISA Write(VISA resource name=w1114, write buffer=w1109, error in (no error)=w1115) -> (error out=w1113:errorcluster)  [unwired: 2 out]
          }
        }
      }
      event "Set temperature (K)": Value Change {
        n553 = event-data() -> ()  [unwired: 1 in, 6 out]
        n554 = local read "Set temperature (K)"() -> (w1121:dbl)
        n555 = Number To Fractional String(number=w1121, precision (6)=i16 3) -> (F-format string=w1124:string)  [unwired: 2 in]
        n556 = Concatenate Strings("SETP 1," ("write buffer"), w1124) -> (w1122:string)
        n557 = VISA Write(VISA resource name=w1118, write buffer=w1122, error in (no error)=w1120) -> (error out=w1119:errorcluster)  [unwired: 2 out]
      }
      event "Temp Ramping Rate (K/min)": Value Change {
        n558 = event-data() -> ()  [unwired: 1 in, 6 out]
        n559 = local read "Temp Ramping Rate (K/min)"() -> (w1128:dbl)
        n560 = Number To Fractional String(number=w1128, precision (6)=i16 1) -> (F-format string=w1134:string)  [unwired: 2 in]
        n561 = Concatenate Strings("RAMP 1,1," ("string"), w1134) -> (w1133:string)
        n562 = VISA Write(VISA resource name=w1131, write buffer=w1133, error in (no error)=w1130) -> (error out=w1129:errorcluster)  [unwired: 2 out]
      }
      event "Heater Range": Value Change {
        n563 = event-data() -> ()  [unwired: 1 in, 6 out]
        n564 = local read "Heater On/Off"() -> (w1140:bool)
        n565 = case shown="True" w1140 {
          tunnel: w1139 -> [w1141 w1146]
          tunnel: [w1141 w1145] -> w1138
          tunnel: w1136 -> [_ w1144]
          frame False {
          }
          frame True {
            n566 = local read "Heater Range"() -> (w1142:enum16{"Off", "Low", "Medium", "High"})
            n567 = Number To Decimal String(number=w1142) -> (decimal integer string=w1148:string)  [unwired: 1 in]
            n568 = Concatenate Strings("RANGE,1," ("write buffer"), w1148) -> (w1147:string)
            n569 = VISA Write(VISA resource name=w1144, write buffer=w1147, error in (no error)=w1146) -> (error out=w1145:errorcluster)  [unwired: 2 out]
          }
        }
      }
    }
    n570 = Reciprocal(x="Sampling rate (Hz)") -> (1/x=w822:dbl)
    n571 = Multiply(x=w822, y=1000.0) -> (x*y=w820:dbl)
    n572 = Wait Until Next ms Multiple(millisecond multiple=w820) -> ()  [unwired: 1 out]
  }
  n573 = local read "Max Field (T)"() -> (w38:dbl)
  n574 = local read "Min Field (T)"() -> (w40:dbl)
  n575 = local read "dB (T)"() -> (w39:dbl)
  n576 = Divide(x=w38, y=w39) -> (x/y=w41:dbl)
  n577 = for {
    N: w41 -> [_]
    tunnel: w39 -> [w1153]
    tunnel: [w1150] -> w37 mode=indexing
    tunnel: w40 -> [w1151]
    tunnel: [0.0] -> _ mode=indexing
    i -> [w1154]
    n578 = Multiply(x=w1154, y=w1153) -> (x*y=w1152:dbl)
    n579 = Add(x=w1152, y=w1151) -> (x+y=w1150:dbl)
  }
  n580 = local write "B array"(w37) -> ()
  n581 = local read "Lake Shore"() -> (w52:refnum<visa-resource-name>)
  n582 = local read "IV converter"() -> (w69:refnum<visa-resource-name>)
  n583 = local read "Magnetic Field"() -> (w68:refnum<visa-resource-name>)
  n584 = VISA Close(VISA resource name=w69, error in (no error)=w71) -> (error out=w72:errorcluster)
  n585 = VISA Close(VISA resource name=w68, error in (no error)=w72) -> (error out=w70:errorcluster)
  n586 = Release Queue(queue=w78, error in (no error)=w70) -> (error out=w65:errorcluster)  [unwired: 1 in, 2 out]
  n587 = Merge Errors(w65, w64) -> (w66:errorcluster)
  n588 = VISA Close(VISA resource name=w52, error in (no error)=w66) -> (error out=w63:errorcluster)
  n589 = local read "refnum out"() -> (w61:refnum<file>)
  n590 = Close File(refnum=w61, error in=w63) -> (error out=w62:errorcluster)  [unwired: 1 out]
  n591 = call <vilib>:"Simple Error Handler.vi"("error in (no error)"=w62) -> ()  [unwired: 4 in, 5 out]
  "i" <- w30
  "j" <- w30
